vi "svx_Timebase Property Dialog.vi"(0 "Container":refnum<vi>, 1 "Data":T2, 2 "State in":T4={"X Scale"={"Name"="Time", "FString"="%#.2g", "Major Color"=16777238, "Minor Color"=16777216, "Grid Style"=1, "Maximum"=0.5, "Minimum"=0.0, "Autoscale"=TRUE, "Show Scale Label"={"Probe X"=FALSE, "Probe Y"=TRUE}, "Show Scale"={"Probe X"=TRUE, "Probe Y"=TRUE}, "Autoscale Once"=FALSE}, "Y Scale"={"Name"="Amplitude", "FString"="%#.2g", "Major Color"=16777238, "Minor Color"=16777216, "Scale Visible"=TRUE, " Label Visible"=TRUE, "Grid Style"=1, "Autoscale"=TRUE, "Maximum"={"Probe X"=1.0, "Probe Y"=1.0}, "Minimum"={"Probe X"=-1.0, "Probe Y"=-1.0}, "Autoscale Once"=FALSE}, "Plot"={"Point Style"=0, "Line Width"=0, "Line Style"=0, "Plot Color"=16860, "Point/fill"=16860}, "Tacho Point Color"=16711680, "Property Name"=[], "Container Bounds"={"Width"=640, "Height"=360}, "Background color"=16777226, "Legend Visible"=TRUE, "Scale Range Change"=refnum, "Strings[]"={"Custom pair name"=FALSE, "Row Strings []"=[], "Column Strings []"=[]}, "Cursor"={"Cursor Point Style"=13, "Cursor Style"=5, "Cursor Line Width"=1, "Cursor Line Style"=0, "Cursor Color"=16860, "Cursor Name Visible"=TRUE, "Cursor Visible"=TRUE, "Cursor Lock"=FALSE, "Cursor Index"=0}, "Index"=[], "Legend Width"=200, " Parents Tags"=[], "Children Tags"=[], "Open?"=[], "Label"="Timebase Plot", "Cursor X Pos"={"X"=0.0, "Y"=0.0}, "Cursor Y Pos"={"X"=0.0, "Y"=0.0}, "Graph Type"=enum."Probe X and Y", "Prev Graph Type"=enum."Probe X and Y", "Prev Legend Visible"=TRUE, "Cursor Release"=refnum, "Pair Strings Changed?"=FALSE, "Cursor ID"=refnum, "Legend Background"=16777226, "Legend Font"=16777222, "Probe Y Label"="Probe Y", "Probe X Label"="Probe X", "Probe X Label Visible"=TRUE, "Probe Y Label Visible"=TRUE, "Tree Item Width"=200, "# Custom RowStr"=0, "# Custom ColStr"=0, "Property Name"=refnum, "Data Related State"=refnum} caption="State", 5 "Ref Ins":T1, 7 "Facade VI":refnum<vi>, 13 "Action in":T3 caption="Action") -> (3 "State out":T4={"X Scale"={"Name"="Time", "FString"="%#.2g", "Major Color"=16777238, "Minor Color"=16777216, "Grid Style"=1, "Maximum"=0.5, "Minimum"=0.0, "Autoscale"=TRUE, "Show Scale Label"={"Probe X"=FALSE, "Probe Y"=TRUE}, "Show Scale"={"Probe X"=TRUE, "Probe Y"=TRUE}, "Autoscale Once"=FALSE}, "Y Scale"={"Name"="Amplitude", "FString"="%#.2g", "Major Color"=16777238, "Minor Color"=16777216, "Scale Visible"=TRUE, " Label Visible"=TRUE, "Grid Style"=1, "Autoscale"=TRUE, "Maximum"={"Probe X"=1.0, "Probe Y"=1.0}, "Minimum"={"Probe X"=-1.0, "Probe Y"=-1.0}, "Autoscale Once"=FALSE}, "Plot"={"Point Style"=0, "Line Width"=0, "Line Style"=0, "Plot Color"=16860, "Point/fill"=16860}, "Tacho Point Color"=16711680, "Property Name"=[], "Container Bounds"={"Width"=640, "Height"=360}, "Background color"=16777226, "Legend Visible"=TRUE, "Scale Range Change"=refnum, "Strings[]"={"Custom pair name"=FALSE, "Row Strings []"=[], "Column Strings []"=[]}, "Cursor"={"Cursor Point Style"=13, "Cursor Style"=5, "Cursor Line Width"=1, "Cursor Line Style"=0, "Cursor Color"=16860, "Cursor Name Visible"=TRUE, "Cursor Visible"=TRUE, "Cursor Lock"=FALSE, "Cursor Index"=0}, "Index"=[], "Legend Width"=200, " Parents Tags"=[], "Children Tags"=[], "Open?"=[], "Label"="Timebase Plot", "Cursor X Pos"={"X"=0.0, "Y"=0.0}, "Cursor Y Pos"={"X"=0.0, "Y"=0.0}, "Graph Type"=enum."Probe X and Y", "Prev Graph Type"=enum."Probe X and Y", "Prev Legend Visible"=TRUE, "Cursor Release"=refnum, "Pair Strings Changed?"=FALSE, "Cursor ID"=refnum, "Legend Background"=16777226, "Legend Font"=16777222, "Probe Y Label"="Probe Y", "Probe X Label"="Probe X", "Probe X Label Visible"=TRUE, "Probe Y Label Visible"=TRUE, "Tree Item Width"=200, "# Custom RowStr"=0, "# Custom ColStr"=0, "Property Name"=refnum, "Data Related State"=refnum} caption="State", 14 "Action out":T3 caption="Action")   [LabVIEW 2017, in "SVX Timebase.xctl"]
uses:
  <vilib>/addons/_XControls/Timebase Plot/SVX Timebase.xctl
  <vilib>/addons/_XControls/Timebase Plot/subVIs/svx_Timebase State.ctl
  <vilib>/addons/_XControls/Timebase Plot/subVIs/svx_Timebase Bounds.ctl
  <vilib>/addons/_XControls/Timebase Plot/subVIs/svx_Timebase Graph Types.ctl
  <vilib>/addons/_XControls/Timebase Plot/subVIs/svx_Timebase Data Related State.ctl
  <vilib>/_xctls/Action.ctl
  <vilib>/addons/_XControls/Timebase Plot/subVIs/svx_Timebase Data.ctl
  <vilib>/addons/_XControls/Timebase Plot/subVIs/svx_Timebase Core States.ctl
  <vilib>/_xctls/XControlSupport.lvlib
panel:
  in  "Help":bool
  in  "Cancel":bool
  in  "OK":bool
  in  "Main Tab":T8(tab)
  in  "Legend Font.Color":u32(colorbox)=16777222 caption="Legend font"
  in  "Legend Background.Color":u32(colorbox)=16777226 caption="Legend background"
  in  "Probe Y Label.Visible":bool=TRUE caption="Probe Y Visible"
  in  "Probe Y Label.Text":string="Probe Y"
  in  "Probe X Label.Visible":bool=TRUE caption="Probe X"
  in  "Probe X Label.Text":string="Probe X"
  in  "Background.Color":u32(colorbox)=16777226 caption="Background"
  in  "Label.Visible":bool=TRUE
  in  "Label.Text":string="Timebase Plot"
  in  "Caption.Visible":bool
  in  "Caption.Text":string="Timebase Plot"
  in  "Enable State":T9(radio)
  in  "Format Selection":u16(ring) items=["Time (X-Axis)", "Amplitude (Y-Axis)"]
  in  "Hide trailing zeros":bool=TRUE
  in  "Digits":u8=2
  in  "Precision Type":u16(ring) items=["Digits of precision", "Significant digits"]
  in  "Type":i32(listbox)=2
  in  "Point/Fill.Color":u32(colorbox) caption="Point/Fill"
  in  "Plot.Point Style":T10={"OK Button 17"=TRUE, "OK Button"=FALSE, "OK Button 2"=FALSE, "OK Button 3"=FALSE, "OK Button 4"=FALSE, "OK Button 5"=FALSE, "OK Button 6"=FALSE, "OK Button 7"=FALSE, "OK Button 8"=FALSE, "OK Button 9"=FALSE, "OK Button 10"=FALSE, "OK Button 11"=FALSE, "OK Button 12"=FALSE, "OK Button 13"=FALSE, "OK Button 14"=FALSE, "OK Button 15"=FALSE, "OK Button 16"=FALSE} caption="Point Style"
  in  "Line.Color":u32(colorbox)=9727 caption="Line"
  in  "Plot.Line Style":T11={"OK Button"=TRUE, "OK Button 2"=FALSE, "OK Button 3"=FALSE, "OK Button 4"=FALSE, "OK Button 5"=FALSE} caption="Line Style"
  in  "Plot.Line Width":T12={"OK Button 2"=TRUE, "OK Button 3"=FALSE, "OK Button 4"=FALSE, "OK Button 5"=FALSE, "OK Button 6"=FALSE, "OK Button 7"=FALSE} caption="Line Width"
  in  "Trigger Point.Color":u32(colorbox)=16711680 caption="Trigger point"
  in  "X Axis Scale":T13={"Probe Y Scale.Visible"=TRUE, "Probe Y Scale Label.Visible"=TRUE, "Probe X Scale.Visible"=TRUE, "Probe X Scale Label.Visible"=TRUE}
  in  "X Axis Range":cluster{"Minimum X":dbl, "Maximum X":dbl}={"Minimum X"=0.0, "Maximum X"=0.5} {"Maximum X" format="%#.6g"; "Minimum X" format="%#.6g"}
  in  "Y Axis Scale":T14={"Scale Visible"=TRUE, "Scale Label Visible"=TRUE}
  in  "Y Axis Range":T15={"Minimum Y [Probe X]"=0.0, "Maximum Y [Probe X]"=10.0, "Minimum Y [Probe Y]"=0.0, "Maximum Y [Probe Y]"=10.0} {"Maximum Y [Probe Y]" format="%#.6g"; "Minimum Y [Probe Y]" format="%#.6g"; "Maximum Y [Probe X]" format="%#.6g"; "Minimum Y [Probe X]" format="%#.6g"}
  in  "YGrid Style":u16(ring) caption="Grid Style and Colors"
  in  "XGrid Style":u16(ring)=1 caption="Grid Style and Colors"
  in  "Minor Grid.Color":u32(colorbox)=16777216 caption="Minor grid"
  in  "Major Grid.Color":u32(colorbox)=16777238 caption="Major grid"
  in  "Scale Fit":bool=TRUE caption="Autoscale"
  in  "Scale Name":string="Time" caption="Name"
  in  "Scale Selection":u16(ring) items=["Time (X-Axis)", "Amplitude (Y-Axis)"]
  in  "Cursor Info Position.Lock":bool
  in  "Cursor.Line Width":T12={"OK Button 2"=FALSE, "OK Button 3"=TRUE, "OK Button 4"=FALSE, "OK Button 5"=FALSE, "OK Button 6"=FALSE, "OK Button 7"=FALSE} caption="Cursor Line Width"
  in  "Cursor.Point Style":T10={"OK Button 17"=FALSE, "OK Button"=FALSE, "OK Button 2"=FALSE, "OK Button 3"=FALSE, "OK Button 4"=FALSE, "OK Button 5"=FALSE, "OK Button 6"=FALSE, "OK Button 7"=FALSE, "OK Button 8"=FALSE, "OK Button 9"=FALSE, "OK Button 10"=FALSE, "OK Button 11"=FALSE, "OK Button 12"=FALSE, "OK Button 13"=TRUE, "OK Button 14"=FALSE, "OK Button 15"=FALSE, "OK Button 16"=FALSE} caption="Cursor Point Style"
  in  "Cursor.Line Style":T11={"OK Button"=TRUE, "OK Button 2"=FALSE, "OK Button 3"=FALSE, "OK Button 4"=FALSE, "OK Button 5"=FALSE} caption="Cursor Line Style"
  in  "Cursor Info.Visible":bool=TRUE caption="Show name"
  in  "Cursor.Style":T16={"OK Button 17"=FALSE, "OK Button"=FALSE, "OK Button 2"=FALSE, "OK Button 5"=FALSE, "OK Button 13"=FALSE, "OK Button 10"=TRUE, "OK Button 6"=FALSE, "OK Button 9"=FALSE, "OK Button 14"=FALSE} caption="Cursor Style"
  in  "Cursor.Color":u32(colorbox)=9727 caption="Cursor color"
  in  "Cursor.Visible":bool=TRUE
  in  "Tip strip":string
  in  "Description":string
  # "Label"
  # "Caption"
  # "Probe X Label"
  # "Probe Y Label"
  # "Color Scheme"
  # "Enabled State"
  # "Timebase Plot"
  # "Colors"
  # "Cursor"
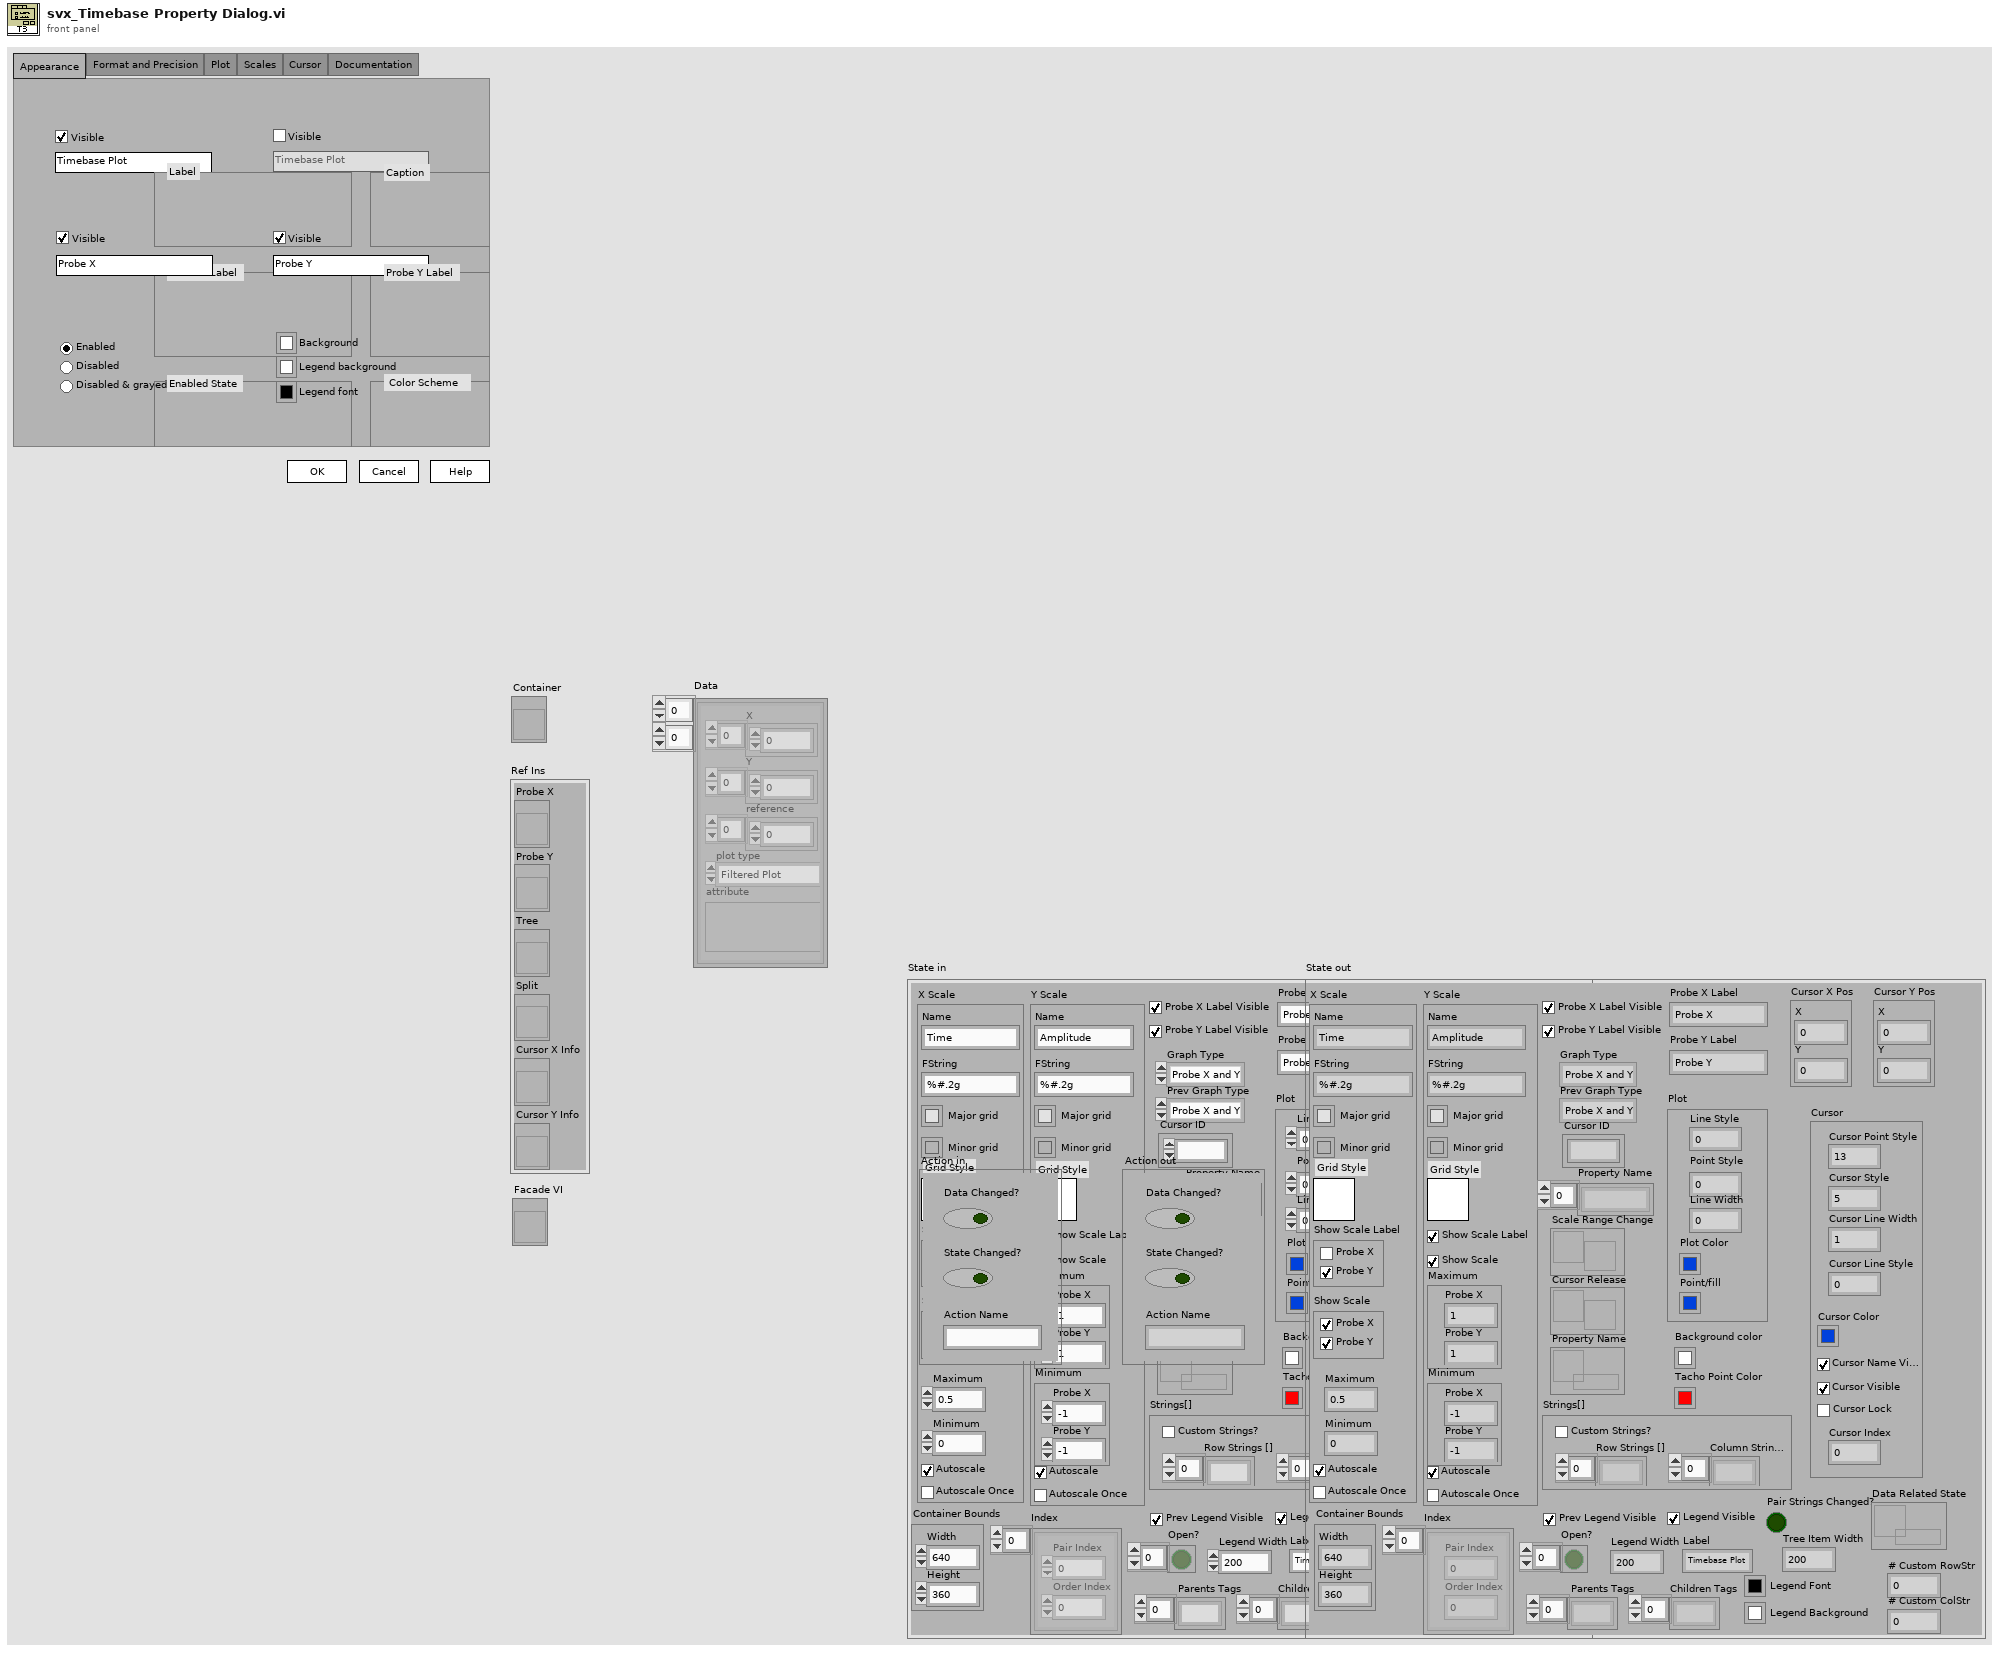
[diagram p1: front panel]
types:
  T1 = cluster{"Probe X":refnum<vi>, "Probe Y":refnum<vi>, "Tree":refnum<vi>, "Split":refnum<vi>, "Cursor X Info":refnum<vi>, "Cursor Y Info":refnum<vi>}
  T2 = typedef "SVX Timebase.xctl/svx_Timebase Data.ctl" = cluster{"X":dbl[], "Y":dbl[], "reference":dbl[], "plot type":enum16{"Filtered Plot", "Unfiltered Plot"}, "attribute":variant}[][]
  T3 = typedef "XControlSupport.lvlib/Action.ctl" = cluster{"Data Changed?":bool, "State Changed?":bool, "Action Name":string}
  T4 = typedef "SVX Timebase.xctl/svx_Timebase State.ctl" = cluster{"X Scale":cluster{"Name":string, "FString":string, "Major Color":u32, "Minor Color":u32, "Grid Style":u16, "Maximum":dbl, "Minimum":dbl, "Autoscale":bool, "Show Scale Label":cluster{"Probe X":bool, "Probe Y":bool}, "Show Scale":cluster{"Probe X":bool, "Probe Y":bool}, "Autoscale Once":bool}, "Y Scale":cluster{"Name":string, "FString":string, "Major Color":u32, "Minor Color":u32, "Scale Visible":bool, " Label Visible":bool, "Grid Style":u16, "Autoscale":bool, "Maximum":cluster{"Probe X":dbl, "Probe Y":dbl}, "Minimum":cluster{"Probe X":dbl, "Probe Y":dbl}, "Autoscale Once":bool}, "Plot":cluster{"Point Style":u8, "Line Width":u8, "Line Style":u8, "Plot Color":u32, "Point/fill":u32}, "Tacho Point Color":u32, "Property Name":string[], "Container Bounds":T5, "Background color":u32, "Legend Visible":bool, "Scale Range Change":refnum<user-event>, "Strings[]":cluster{"Custom pair name":bool, "Row Strings []":string[], "Column Strings []":string[]}, "Cursor":cluster{"Cursor Point Style":u8, "Cursor Style":u8, "Cursor Line Width":u8, "Cursor Line Style":u8, "Cursor Color":u32, "Cursor Name Visible":bool, "Cursor Visible":bool, "Cursor Lock":bool, "Cursor Index":i32}, "Index":cluster{"Pair Index":u32, "Order Index":u32}[], "Legend Width":u32, " Parents Tags":string[], "Children Tags":string[], "Open?":bool[], "Label":string, "Cursor X Pos":cluster{"X":dbl, "Y":dbl}, "Cursor Y Pos":cluster{"X":dbl, "Y":dbl}, "Graph Type":T6, "Prev Graph Type":T6, "Prev Legend Visible":bool, "Cursor Release":refnum<user-event>, "Pair Strings Changed?":bool, "Cursor ID":refnum<k1>, "Legend Background":u32, "Legend Font":u32, "Probe Y Label":string, "Probe X Label":string, "Probe X Label Visible":bool, "Probe Y Label Visible":bool, "Tree Item Width":u32, "# Custom RowStr":u32, "# Custom ColStr":u32, "Property Name":refnum<queue>, "Data Related State":T7}
  T5 = typedef "SVX Timebase.xctl/svx_Timebase Bounds.ctl" = cluster{"Width":u32, "Height":u32}
  T6 = typedef "SVX Timebase.xctl/svx_Timebase Graph Types.ctl" = enum16{"Probe X", "Probe Y", "Probe X and Y"}
  T7 = typedef "SVX Timebase.xctl/svx_Timebase Data Related State.ctl" = refnum<queue>
  T8 = enum32{"Appearance", "Format and Precision", "Plot", "Scales", "Cursor", "Documentation"}
  T9 = enum32{"Enabled", "Disabled", "Disabled & grayed"}
  T10 = cluster{"OK Button 17":bool, "OK Button":bool, "OK Button 2":bool, "OK Button 3":bool, "OK Button 4":bool, "OK Button 5":bool, "OK Button 6":bool, "OK Button 7":bool, "OK Button 8":bool, "OK Button 9":bool, "OK Button 10":bool, "OK Button 11":bool, "OK Button 12":bool, "OK Button 13":bool, "OK Button 14":bool, "OK Button 15":bool, "OK Button 16":bool}
  T11 = cluster{"OK Button":bool, "OK Button 2":bool, "OK Button 3":bool, "OK Button 4":bool, "OK Button 5":bool}
  T12 = cluster{"OK Button 2":bool, "OK Button 3":bool, "OK Button 4":bool, "OK Button 5":bool, "OK Button 6":bool, "OK Button 7":bool}
  T13 = cluster{"Probe Y Scale.Visible":bool, "Probe Y Scale Label.Visible":bool, "Probe X Scale.Visible":bool, "Probe X Scale Label.Visible":bool}
  T14 = cluster{"Scale Visible":bool, "Scale Label Visible":bool}
  T15 = cluster{"Minimum Y [Probe X]":dbl, "Maximum Y [Probe X]":dbl, "Minimum Y [Probe Y]":dbl, "Maximum Y [Probe Y]":dbl}
  T16 = cluster{"OK Button 17":bool, "OK Button":bool, "OK Button 2":bool, "OK Button 5":bool, "OK Button 13":bool, "OK Button 10":bool, "OK Button 6":bool, "OK Button 9":bool, "OK Button 14":bool}
  T17 = cluster{"Desc":string, "TipStrip":string, "Label.Text":string, "Label.Visible":bool, "Caption.Text":string, "Caption.Visible":bool, "Disabled":u8}
  T18 = cluster{"X":dbl[], "Y":dbl[], "reference":dbl[], "plot type":enum16{"Filtered Plot", "Unfiltered Plot"}, "attribute":variant}
  T19 = typedef "SVX Timebase.xctl/svx_Timebase Core States.ctl" = enum16{"None", "[Axis] Range X Scale", "[Axis] Range Y Scale", "[Layout] Graph Type Change", "[Plot] Tacho Point", "[Plot] Grid and BG", "[Cursor] Cursor Info", "[Legend] Pair Strings", "[Data] Plot Data", "[Legend] Checkbox", "[Layout] Update", "[Legend] Tree Open", "[Layout] Legend Visible Change", "[Plot] Data Point", "[Cursor] Appearance", "[Cursor] Index", "[Legend] Color", "[Axis] Axis and Label", "[Axis] Format String", "[Layout] Min Pane Size", "[Data] Index", "[Plot] Caption", "[Data] Legend Strings"}
  T20 = cluster{"Probe X":dbl, "Probe X":dbl, "Probe Y":dbl, "Probe Y":dbl}
  T21 = cluster{"Scale Visible":bool, " Label Visible":bool}
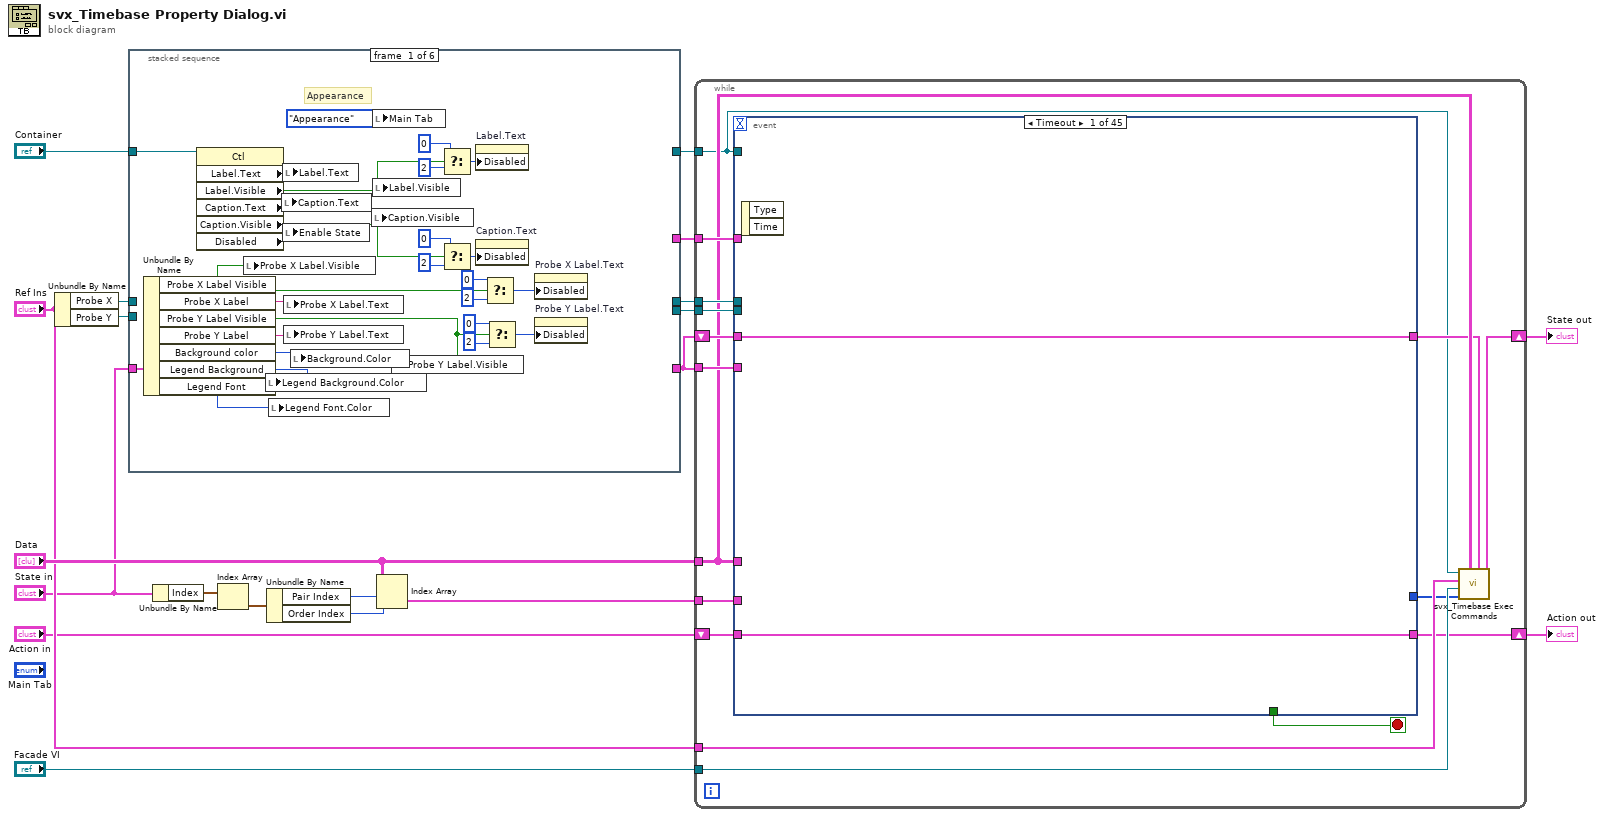
[diagram p0: block diagram]
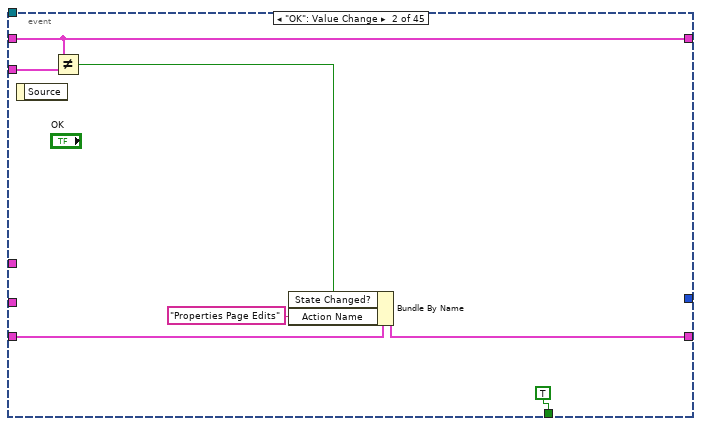
[diagram p2: hidden frame]
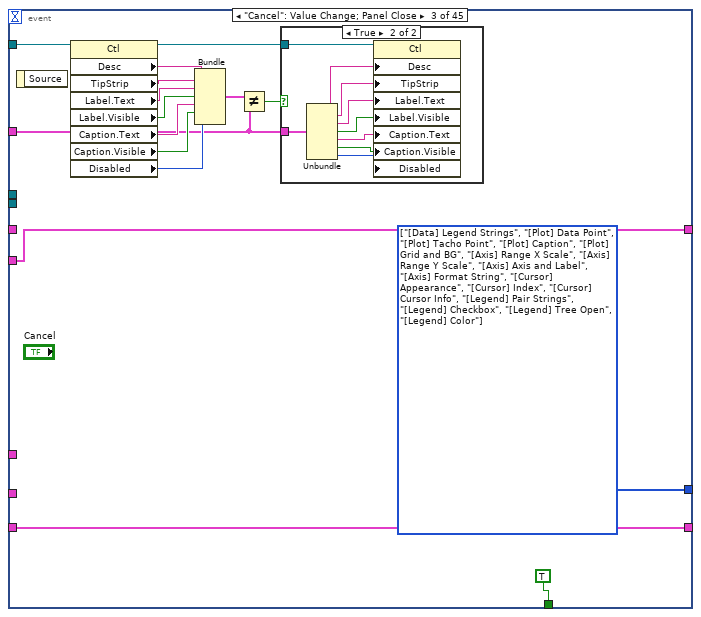
[diagram p3: hidden frame]
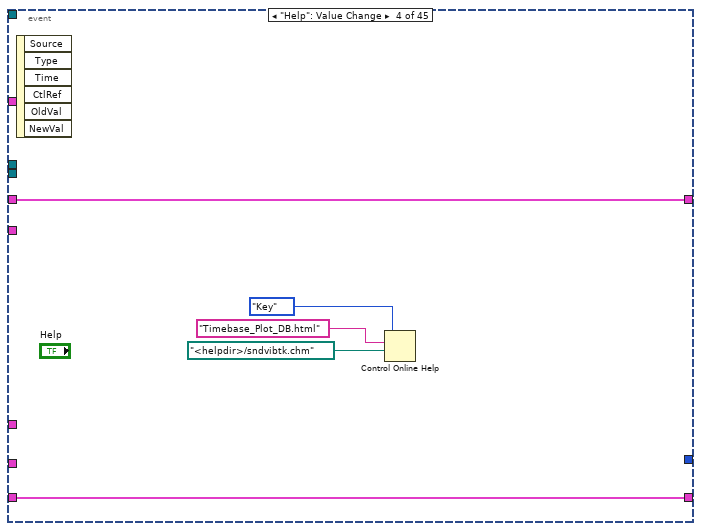
[diagram p5: hidden frame]
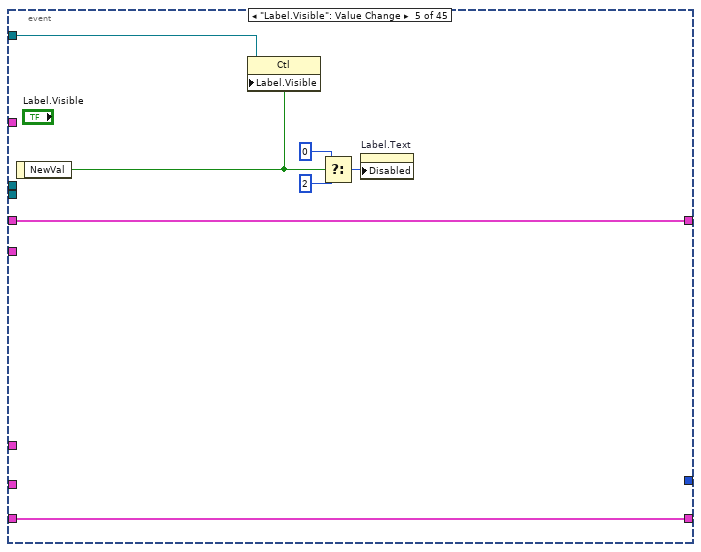
[diagram p6: hidden frame]
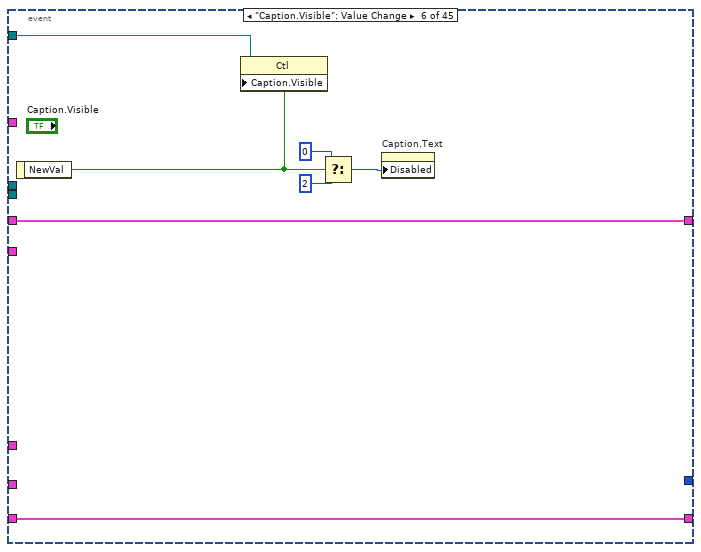
[diagram p7: hidden frame]
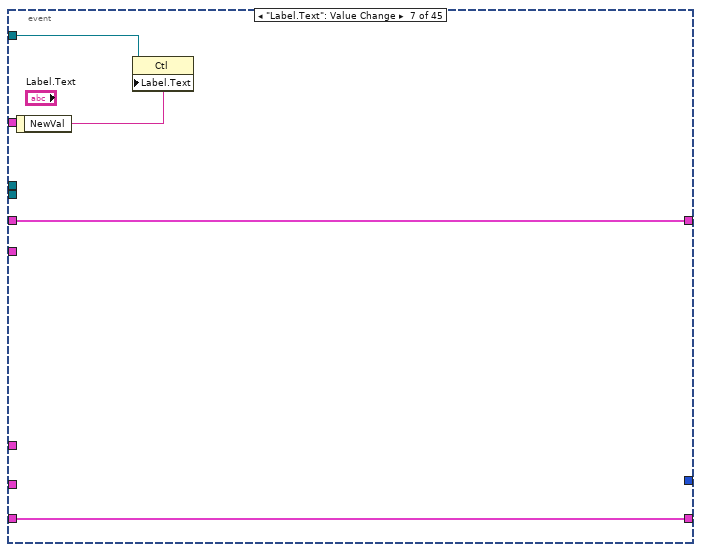
[diagram p8: hidden frame]
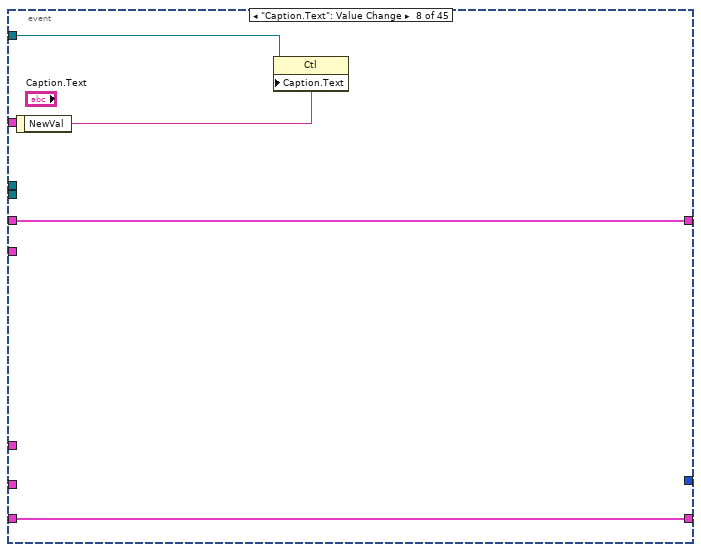
[diagram p9: hidden frame]
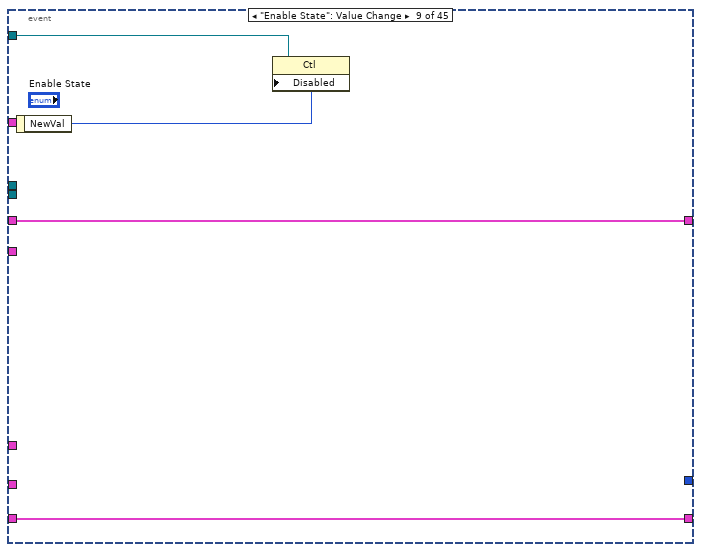
[diagram p10: hidden frame]
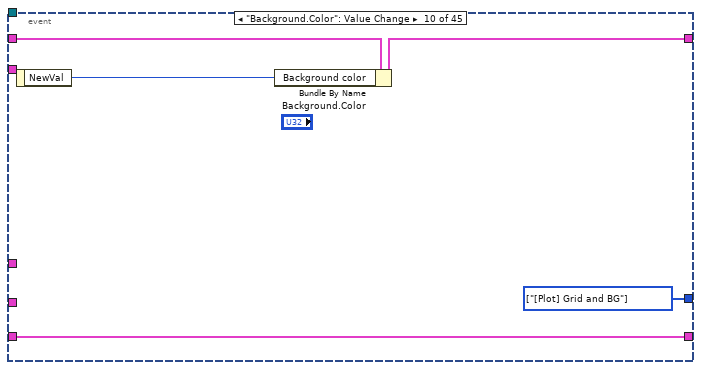
[diagram p11: hidden frame]
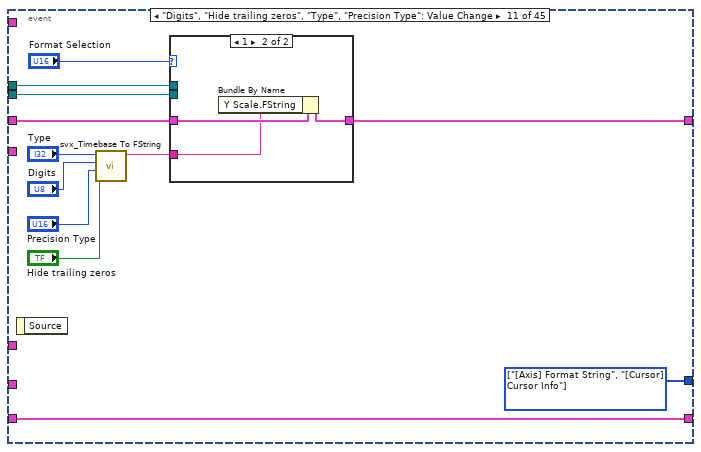
[diagram p12: hidden frame]
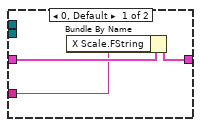
[diagram p13: hidden frame]
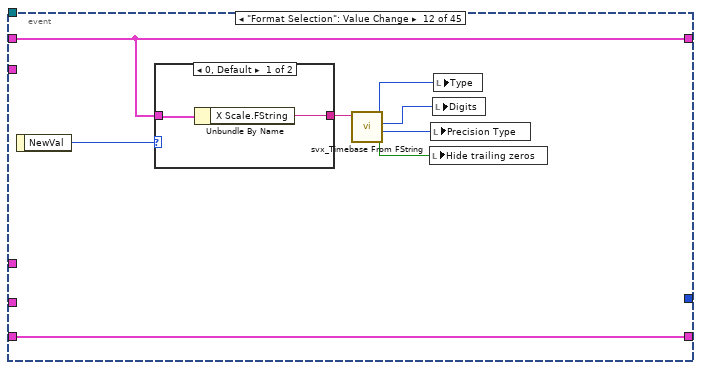
[diagram p14: hidden frame]
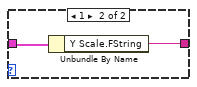
[diagram p15: hidden frame]
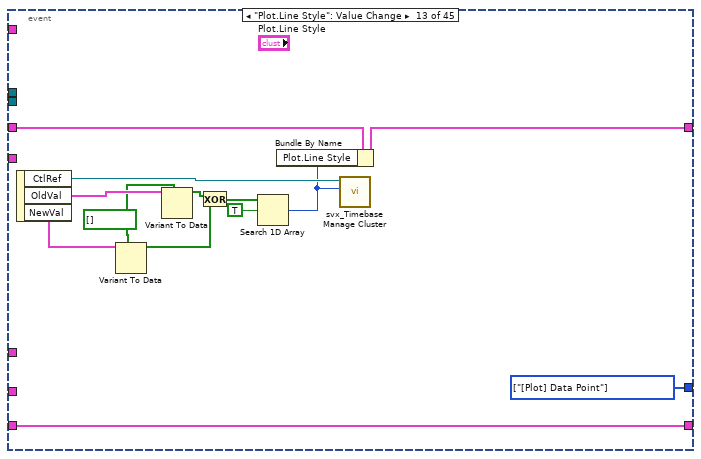
[diagram p16: hidden frame]
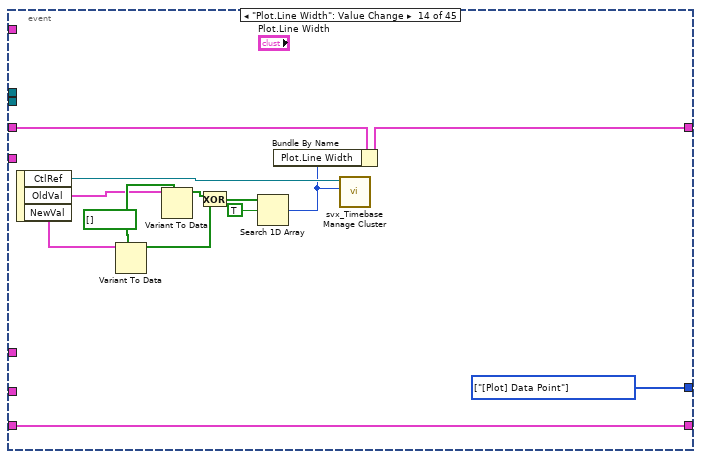
[diagram p17: hidden frame]
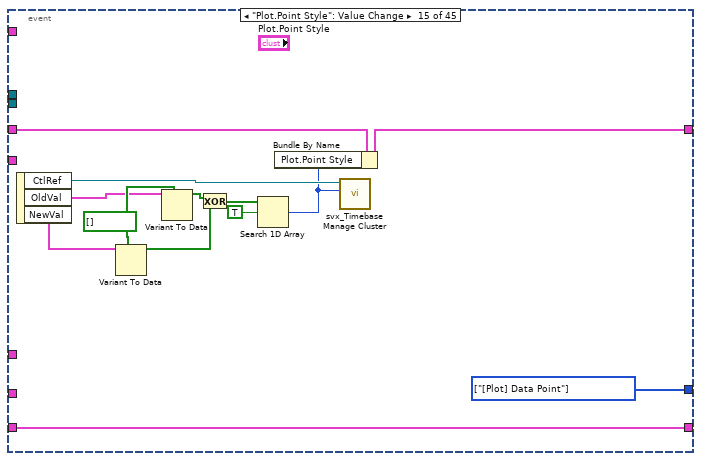
[diagram p18: hidden frame]
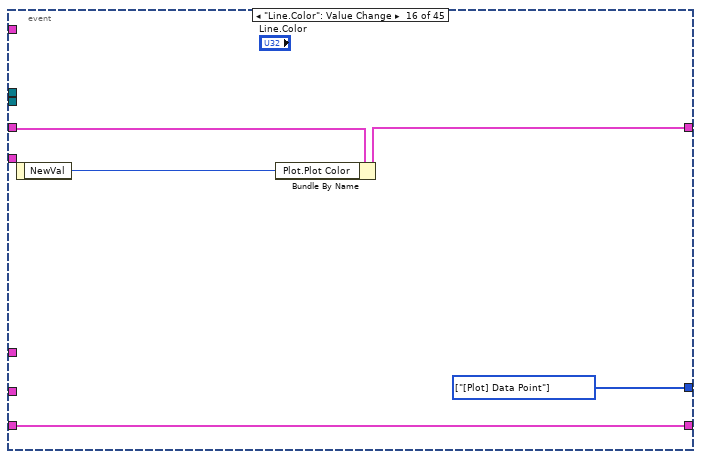
[diagram p19: hidden frame]
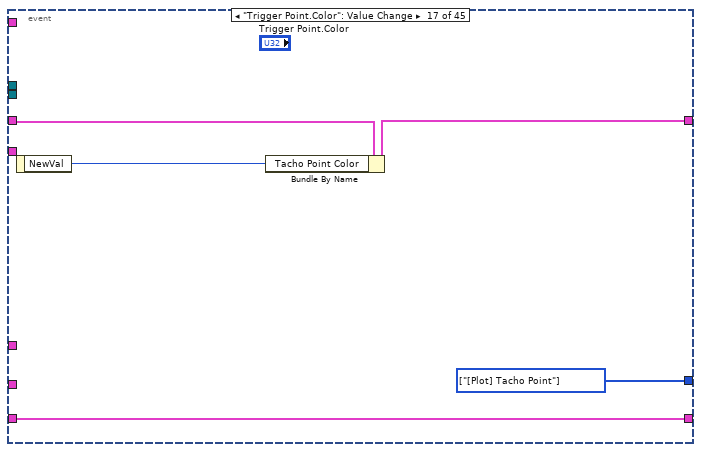
[diagram p20: hidden frame]
diagram:
  n1 = Unbundle By Name("Ref Ins") -> ("Probe X"=w6:refnum<vi>, "Probe Y"=w5:refnum<vi>)
  n2 = stacked-sequence {
    tunnel: "Container" -> [w47 _ _ _ _ w145]
    tunnel: "State in" -> [w45 w60 w74 w101 w132 w135]
    tunnel: [_ _ _ _ _ w144] -> w19
    tunnel: [_ _ _ _ _ w135] -> w18
    tunnel: [_ _ _ _ _ w134] -> w16
    tunnel: w6 -> [_ _ _ _ _ w134]
    tunnel: [_ _ _ _ _ w136] -> w15
    tunnel: w5 -> [_ _ _ _ _ w133]
    tunnel: [_ _ _ _ _ w133] -> w7
    frame #0 {
      # "Appearance"
      n3 = Unbundle By Name(w45) -> ("Probe X Label Visible"=w28:bool, "Probe X Label"=w32:string, "Probe Y Label Visible"=w24:bool, "Probe Y Label"=w31:string, "Background color"=w46:u32, "Legend Background"=w22:u32, "Legend Font"=w21:u32)
      n4 = property class="Ctl"(reference=w47) -> ("Label.Text"=w39:string, "Label.Visible"=w38:bool, "Caption.Text"=w37:string, "Caption.Visible"=w35:bool, "Disabled"=w36:u8)  [unwired: 1 in, 2 out]
      n5 = local write "Probe X Label.Visible"(w28) -> ()
      n6 = local write "Legend Background.Color"(w22) -> ()
      n7 = local write "Legend Font.Color"(w21) -> ()
      n8 = local write "Caption.Text"(w37) -> ()
      n9 = local write "Label.Text"(w39) -> ()
      n10 = local write "Enable State"(w36) -> ()
      n11 = local write "Probe X Label.Text"(w32) -> ()
      n12 = local write "Probe Y Label.Text"(w31) -> ()
      n13 = local write "Background.Color"(w46) -> ()
      n14 = local write "Caption.Visible"(w35) -> ()
      n15 = local write "Main Tab"(T8."Appearance" ("Main Tab")) -> ()
      n16 = local write "Label.Visible"(w38) -> ()
      n17 = local write "Probe Y Label.Visible"(w24) -> ()
      n18 = Select(t=u8 0 ("Disabled"), s=w38, f=u8 2) -> (s? t:f=w43:u8)
      n19 = Select(t=u8 0 ("Disabled"), s=w35, f=u8 2) -> (s? t:f=w40:u8)
      n20 = property on="Label.Text" class="Str"("Disabled"=w43) -> ()  [unwired: 2 in, 2 out]
      n21 = property on="Caption.Text" class="Str"("Disabled"=w40) -> ()  [unwired: 2 in, 2 out]
      n22 = Select(t=u8 0 ("Disabled"), s=w28, f=u8 2) -> (s? t:f=w27:u8)
      n23 = Select(t=u8 0 ("Disabled"), s=w24, f=u8 2) -> (s? t:f=w23:u8)
      n24 = property on="Probe X Label.Text" class="Str"("Disabled"=w27) -> ()  [unwired: 2 in, 2 out]
      n25 = property on="Probe Y Label.Text" class="Str"("Disabled"=w23) -> ()  [unwired: 2 in, 2 out]
    }
    frame #1 {
      w61 = u16 0 items=["X-Axis", "Y-Axis"] ("Format selection")
      # "On Tab 3"
      # "Format and Precision"
      n26 = Unbundle By Name(w60) -> ("X Scale.Name"=w54:string, "Y Scale.Name"=w51:string, "X Scale.FString"=w59:string)
      n27 = call <vilib>:"svx_Timebase From FString.vi"("Format string"=w59) -> ("trailing zeros"=w55:bool, "Precision Type"=w56:u16, "Digits"=w57:u8, "Type"=w58:i32)  [unwired: 7 in]
      n28 = local write "Format Selection"(w61) -> ()
      n29 = Concatenate Strings(w54, " (X-Axis)" ("string")) -> (w50:string)
      n30 = Concatenate Strings(w51, " (Y-Axis)" ("string")) -> (w49:string)
      n31 = local write "Hide trailing zeros"(w55) -> ()
      n32 = local write "Precision Type"(w56) -> ()
      n33 = local write "Digits"(w57) -> ()
      n34 = local write "Type"(w58) -> ()
      n35 = Build Array(w50, w49) -> (w48:string[])
      n36 = property on="Format Selection" class="Ring (strict)"("Strings []"=w48) -> ()  [unwired: 2 in, 2 out]
      n37 = property on="Scale Selection" class="Ring (strict)"("Strings []"=w48) -> ()  [unwired: 2 in, 2 out]
    }
    frame #2 {
      # "Plot"
      n38 = Unbundle By Name(w74) -> ("Plot.Plot Color"=w67:u32, "Tacho Point Color"=w66:u32, "Plot.Point/fill"=w65:u32, "Plot.Line Width"=w73:u8, "Plot.Line Style"=w71:u8, "Plot.Point Style"=w70:u8)
      n39 = control-ref of="Plot.Line Width"() -> (w72:refnum<vi>)
      n40 = control-ref of="Plot.Line Style"() -> (w68:refnum<vi>)
      n41 = control-ref of="Plot.Point Style"() -> (w69:refnum<vi>)
      n42 = To Long Integer(number=w73) -> (32bit integer=w64:i32)
      n43 = To Long Integer(number=w71) -> (32bit integer=w63:i32)
      n44 = To Long Integer(number=w70) -> (32bit integer=w62:i32)
      n45 = local write "Point/Fill.Color"(w65) -> ()
      n46 = local write "Trigger Point.Color"(w66) -> ()
      n47 = local write "Line.Color"(w67) -> ()
      n48 = call <vilib>:"svx_Timebase Manage Cluster.vi"("index"=w64, "Cursor Refnum"=w72) -> ()  [unwired: 10 in]
      n49 = call <vilib>:"svx_Timebase Manage Cluster.vi"("index"=w63, "Cursor Refnum"=w68) -> ()  [unwired: 10 in]
      n50 = call <vilib>:"svx_Timebase Manage Cluster.vi"("index"=w62, "Cursor Refnum"=w69) -> ()  [unwired: 10 in]
    }
    frame #3 {
      w102 = u16 0 items=["X-Axis", "Y-Axis"] ("Scale selection")
      # "Scales"
      n51 = Unbundle By Name(w101) -> ("X Scale.Name"=w100:string, "X Scale.Show Scale.Probe X"=w78:bool, "X Scale.Show Scale Label.Probe X"=w77:bool, "X Scale.Show Scale.Probe Y"=w76:bool, "X Scale.Show Scale Label.Probe Y"=w75:bool, "X Scale.Grid Style"=w91:u16, "X Scale.Major Color"=w99:u32, "X Scale.Minor Color"=w98:u32, "X Scale.Autoscale"=w95:bool, "X Scale.Minimum"=w87:dbl, "X Scale.Maximum"=w86:dbl)
      n52 = property on="YGrid Style" class="Ring (strict)"("Visible"=FALSE) -> ()  [unwired: 2 in, 2 out]
      n53 = property on="XGrid Style" class="Ring (strict)"("Visible"=TRUE) -> ()  [unwired: 2 in, 2 out]
      n54 = Bundle("Minimum"=w87, "Maximum"=w86) -> (w85:cluster{"Minimum":dbl, "Maximum":dbl})  [unwired: 1 in]
      n55 = local write "X Axis Range"(w85) -> ()
      n56 = local write "Scale Selection"(w102) -> ()
      n57 = local write "Minor Grid.Color"(w98) -> ()
      n58 = local write "XGrid Style"(w91) -> ()
      n59 = case shown="0, Default" w91 {
        tunnel: [w105 u8 0 ("Disabled") w108] -> w93
        tunnel: [w105 u8 2 ("Disabled") w108] -> w92
        frame 0, Default {
          w105 = u8 2 ("Disabled")
        }
        frame 1 {
        }
        frame 2 {
          w108 = u8 0 ("Disabled")
        }
      }
      n60 = local write "Scale Name"(w100) -> ()
      n61 = Select(t=u8 2 ("Disabled"), s=w95, f=u8 0) -> (s? t:f=w83:u8)
      n62 = property on="X Axis Range" class="Clust (strict)"("Disabled"=w83, "Visible"=TRUE) -> ("Controls[]"=w84:refnum<vi>[])  [unwired: 2 in, 2 out]
      n63 = Bundle By Name(cluster=T13 {"Probe Y Scale.Visible"=TRUE, "Probe Y Scale Label.Visible"=TRUE, "Probe X Scale.Visible"=TRUE, "Probe X Scale Label.Visible"=TRUE} ("X Axis Scale"), "Probe X Scale.Visible"=w78, "Probe X Scale Label.Visible"=w77, "Probe Y Scale.Visible"=w76, "Probe Y Scale Label.Visible"=w75) -> (w79:T13)
      n64 = local write "Major Grid.Color"(w99) -> ()
      n65 = local write "Scale Fit"(w95) -> ()
      n66 = property on="Major Grid.Color" class="ColBox"("Disabled"=w93) -> ()  [unwired: 2 in, 2 out]
      n67 = property on="Minor Grid.Color" class="ColBox"("Disabled"=w92) -> ()  [unwired: 2 in, 2 out]
      n68 = for {
        tunnel: w84 -> [w104] mode=indexing
        tunnel: w83 -> [w103]
        n69 = property class="Ctl"(reference=w104, "Disabled"=w103) -> ()  [unwired: 1 in, 2 out]
      }
      n70 = property on="Y Axis Range" class="Clust (strict)"("Visible"=FALSE) -> ()  [unwired: 2 in, 2 out]
      n71 = property on="X Axis Scale" class="Clust (strict)"("Visible"=TRUE) -> ()  [unwired: 2 in, 2 out]
      n72 = property on="Y Axis Scale" class="Clust (strict)"("Visible"=FALSE) -> ()  [unwired: 2 in, 2 out]
      n73 = local write "X Axis Scale"(w79) -> ()
    }
    frame #4 {
      # "Cursor"
      n74 = Unbundle By Name(w132) -> ("Cursor.Cursor Point Style"=w131:u8, "Cursor.Cursor Style"=w129:u8, "Cursor.Cursor Line Width"=w127:u8, "Cursor.Cursor Line Style"=w125:u8, "Cursor.Cursor Color"=w123:u32, "Cursor.Cursor Lock"=w122:bool, "Cursor.Cursor Name Visible"=w115:bool, "Cursor.Cursor Visible"=w114:bool)
      n75 = control-ref of="Cursor.Point Style"() -> (w130:refnum<vi>)
      n76 = local write "Cursor.Visible"(w114) -> ()
      n77 = To Long Integer(number=w131) -> (32bit integer=w109:i32)
      n78 = local write "Cursor Info.Visible"(w115) -> ()
      n79 = local write "Cursor Info Position.Lock"(w122) -> ()
      n80 = call <vilib>:"svx_Timebase Manage Cluster.vi"("index"=w109, "Cursor Refnum"=w130) -> ()  [unwired: 10 in]
      n81 = And(x=w115, y=w114) -> (x .and. y?=w113:bool)
      n82 = To Long Integer(number=w129) -> (32bit integer=w112:i32)
      n83 = To Long Integer(number=w125) -> (32bit integer=w110:i32)
      n84 = control-ref of="Cursor.Style"() -> (w128:refnum<vi>)
      n85 = control-ref of="Cursor.Line Style"() -> (w124:refnum<vi>)
      n86 = local write "Cursor.Color"(w123) -> ()
      n87 = To Long Integer(number=w127) -> (32bit integer=w111:i32)
      n88 = call <vilib>:"svx_Timebase Manage Cluster.vi"("index"=w112, "Cursor Refnum"=w128) -> ()  [unwired: 10 in]
      n89 = call <vilib>:"svx_Timebase Manage Cluster.vi"("index"=w110, "Cursor Refnum"=w124) -> ()  [unwired: 10 in]
      n90 = Select(t=u8 0, s=w113, f=u8 2) -> (s? t:f=w116:u8)
      n91 = Select(t=u8 0, s=w114, f=u8 2) -> (s? t:f=w121:u8)
      n92 = control-ref of="Cursor.Line Width"() -> (w126:refnum<vi>)
      n93 = property on="Cursor Info Position.Lock" class="Bool (strict)"("Disabled"=w116) -> ()  [unwired: 2 in, 2 out]
      n94 = property on="Cursor Info.Visible" class="Bool (strict)"("Disabled"=w121) -> ()  [unwired: 2 in, 2 out]
      n95 = call <vilib>:"svx_Timebase Manage Cluster.vi"("index"=w111, "Cursor Refnum"=w126) -> ()  [unwired: 10 in]
    }
    frame #5 {
      n96 = property class="Ctl"(reference=w145) -> (reference out=w144:refnum<vi>, "Desc"=w137:string, "TipStrip"=w138:string, "Label.Text"=w143:string, "Label.Visible"=w142:bool, "Caption.Text"=w141:string, "Caption.Visible"=w140:bool, "Disabled"=w139:u8)  [unwired: 1 in, 1 out]
      n97 = local write "Description"(w137) -> ()
      n98 = local write "Tip strip"(w138) -> ()
      n99 = Bundle("Desc"=w137, "TipStrip"=w138, "Label.Text"=w143, "Label.Visible"=w142, "Caption.Text"=w141, "Caption.Visible"=w140, "Disabled"=w139) -> (w136:T17)  [unwired: 1 in]
    }
  }
  n100 = Unbundle By Name("State in") -> ("Index"=w11:cluster{"Pair Index":u32, "Order Index":u32}[])
  n101 = Index Array(array=w11) -> (element=w10:cluster{"Pair Index":u32, "Order Index":u32})  [unwired: 1 in]
  n102 = Unbundle By Name(w10) -> ("Pair Index"=w9:u32, "Order Index"=w8:u32)
  n103 = Index Array(array="Data", index (row)=w9, index (col)=w8) -> (element=w12:T18)
  n104 = while {
    tunnel: w19 -> [w149]
    shift-right: [w152] -> w14
    shift-left: w18 -> [w160]
    tunnel: w18 -> [w157]
    tunnel: w16 -> [w159]
    tunnel: w15 -> [w158]
    tunnel: "Data" -> [w154]
    tunnel: w12 -> [w156]
    tunnel: w7 -> [w155]
    tunnel: "Ref Ins" -> [w151]
    tunnel: "Facade VI" -> [w150]
    shift-right: [w146] -> w17
    shift-left: "Action in" -> [w148]
    stop <- w161 stop-if-true
    n105 = event shown="[0] Timeout" {
      selector: _ -> [_ _ _ _ _ _ _ _ _ _ _ _ _ _ _ _ _ _ _ _ _ _ _ _ _ _ _ _ _ _ _ _ _ _ _ _ _ _ _ _ _ _ _ _ _]
      dyn-events: _ -> [_ _ _ _ _ _ _ _ _ _ _ _ _ _ _ _ _ _ _ _ _ _ _ _ _ _ _ _ _ _ _ _ _ _ _ _ _ _ _ _ _ _ _ _ _]
      timeout: _ -> [_ _ _ _ _ _ _ _ _ _ _ _ _ _ _ _ _ _ _ _ _ _ _ _ _ _ _ _ _ _ _ _ _ _ _ _ _ _ _ _ _ _ _ _ _]
      tunnel: [_ TRUE TRUE _ _ _ _ _ _ _ _ _ _ _ _ _ _ _ _ _ _ _ _ _ _ _ _ _ _ _ _ _ _ _ _ _ _ _ _ _ _ _ _ _ _] -> w161
      tunnel: w160 -> [w163 w165 _ w200 w202 w209 w215 w220 w224 w231 w237 w256 w266 w282 w295 w305 w310 w319 w325 w329 w336 w359 w368 w411 w417 w428 w439 w451 w465 w522 w535 w548 w561 w574 w579 w584 w589 w602 w610 w618 w626 w631 w636 w641 w645]
      tunnel: w157 -> [_ w164 w184 _ _ _ _ _ _ _ _ _ _ _ _ _ _ _ _ _ _ _ _ _ _ _ _ _ _ _ _ _ _ _ _ _ _ _ _ _ _ _ _ _ _]
      tunnel: w148 -> [w162 w169 w186 w199 w201 w208 w216 w219 w223 w227 w232 w250 w262 w275 w288 w301 w306 w311 w324 w328 w332 w354 w360 w403 w412 w423 w434 w446 w458 w515 w528 w541 w554 w567 w575 w580 w585 w590 w603 w611 w619 w627 w632 w637 w642]
      tunnel: [w162 w168 w186 w199 w201 w208 w216 w219 w223 w227 w232 w250 w262 w275 w288 w301 w306 w311 w324 w328 w332 w354 w360 w403 w412 w423 w434 w446 w458 w515 w528 w541 w554 w567 w575 w580 w585 w590 w603 w611 w619 w627 w632 w637 w642] -> w146
      tunnel: [_ _ w183 _ _ _ _ _ _ w228 w233 _ w263 w276 w289 w302 w307 w312 _ _ w333 w355 _ w404 w416 w427 w435 w447 _ w516 w529 w542 w555 w568 w576 w581 w586 w591 w604 w612 w620 w628 w633 w638 w643] -> w147
      tunnel: w159 -> [_ _ _ _ _ _ _ _ _ _ w235 _ _ _ _ _ _ _ _ _ _ _ w369 _ _ _ _ _ _ _ _ _ _ _ _ _ _ _ _ _ _ _ _ _ _]
      tunnel: w149 -> [_ _ w182 _ w207 w214 w218 w222 w226 _ _ _ _ _ _ _ _ _ w327 w331 _ _ _ _ _ _ _ _ _ _ _ _ _ _ _ _ _ _ _ _ _ _ _ _ _]
      tunnel: w158 -> [_ _ w172 _ _ _ _ _ _ _ _ _ _ _ _ _ _ _ _ _ _ _ _ _ _ _ _ _ _ _ _ _ _ _ _ _ _ _ _ _ _ _ _ _ _]
      tunnel: [w163 w165 w184 w200 w202 w209 w215 w220 w224 w230 w236 w256 w265 w281 w294 w304 w308 w323 w325 w329 w335 w358 w365 w410 w418 w429 w438 w450 w465 w521 w534 w547 w560 w573 w577 w582 w588 w601 w609 w617 w625 w630 w635 w640 w644] -> w153
      tunnel: w154 -> [_ _ _ _ _ _ _ _ _ _ _ _ _ _ _ _ _ _ _ _ _ _ _ _ _ _ _ _ _ _ _ _ _ _ _ _ _ _ _ _ _ _ _ _ _]
      tunnel: w156 -> [_ _ _ _ _ _ _ _ _ _ _ _ _ _ _ _ _ _ _ _ _ _ w364 _ _ _ _ _ _ _ _ _ _ _ _ _ _ _ _ _ _ _ _ _ _]
      tunnel: w155 -> [_ _ _ _ _ _ _ _ _ _ w234 _ _ _ _ _ _ _ _ _ _ _ w362 _ _ _ _ _ _ _ _ _ _ _ _ _ _ _ _ _ _ _ _ _ _]
      event Timeout {
        n106 = event-data() -> ()  [unwired: 1 in, 2 out]
      }
      event "OK": Value Change {
        n107 = event-data() -> ()  [unwired: 1 in, 1 out]
        n108 = Not Equal?(x=w165, y=w164) -> (x != y?=w167:bool)
        n109 = Bundle By Name(cluster=w169, "State Changed?"=w167, "Action Name"="Properties Page Edits") -> (w168:T3)
      }
      event "Cancel": Value Change; Panel Close {
        w183 = T19[] [enum."[Data] Legend Strings", enum."[Plot] Data Point", enum."[Plot] Tacho Point", enum."[Plot] Caption", enum."[Plot] Grid and BG", enum."[Axis] Range X Scale", enum."[Axis] Range Y Scale", enum."[Axis] Axis and Label", enum."[Axis] Format String", enum."[Cursor] Appearance", enum."[Cursor] Index", enum."[Cursor] Cursor Info", enum."[Legend] Pair Strings", enum."[Legend] Checkbox", enum."[Legend] Tree Open", enum."[Legend] Color"] items=["None", "[Axis] Range X Scale", "[Axis] Range Y Scale", "[Layout] Graph Type Change", "[Plot] Tacho Point", "[Plot] Grid and BG", "[Cursor] Cursor Info", "[Legend] Pair Strings", "[Data] Plot Data", "[Legend] Checkbox", "[Layout] Update", "[Legend] Tree Open", "[Layout] Legend Visible Change", "[Plot] Data Point", "[Cursor] Appearance", "[Cursor] Index", "[Legend] Color", "[Axis] Axis and Label", "[Axis] Format String", "[Layout] Min Pane Size", "[Data] Index", "[Plot] Caption", "[Data] Legend Strings"]
        n110 = event-data() -> ()  [unwired: 1 in, 1 out]
        n111 = property class="Ctl"(reference=w182) -> (reference out=w181:refnum<vi>, "Desc"=w180:string, "TipStrip"=w179:string, "Label.Text"=w178:string, "Label.Visible"=w177:bool, "Caption.Text"=w176:string, "Caption.Visible"=w175:bool, "Disabled"=w174:u8)  [unwired: 1 in, 1 out]
        n112 = Bundle("Desc"=w180, "TipStrip"=w179, "Label.Text"=w178, "Label.Visible"=w177, "Caption.Text"=w176, "Caption.Visible"=w175, "Disabled"=w174) -> (w173:T17)  [unwired: 1 in]
        n113 = Not Equal?(x=w173, y=w172) -> (x != y?=w171:bool)
        n114 = case shown="True" w171 {
          tunnel: w181 -> [_ w188]
          tunnel: w172 -> [_ w187]
          frame False {
          }
          frame True {
            n115 = Unbundle(w187) -> ("Desc"=w195:string, "TipStrip"=w194:string, "Label.Text"=w193:string, "Label.Visible"=w192:bool, "Caption.Text"=w191:string, "Caption.Visible"=w190:bool, "Disabled"=w189:u8)
            n116 = property class="Ctl"(reference=w188, "Desc"=w195, "TipStrip"=w194, "Label.Text"=w193, "Label.Visible"=w192, "Caption.Text"=w191, "Caption.Visible"=w190, "Disabled"=w189) -> ()  [unwired: 1 in, 2 out]
          }
        }
      }
      event "Help": Value Change {
        n117 = event-data() -> ()  [unwired: 1 in, 6 out]
        n118 = Control Online Help(2:path "<helpdir>/sndvibtk.chm" ("Path to the help file"), 3:"Timebase_Plot_DB.html" ("String to search for"), 4:enum16{"Contents", "Key", "Close"}."Key" ("Operation")) -> ()  [unwired: 1 in, 1 out]
      }
      event "Label.Visible": Value Change {
        n119 = event-data() -> ("NewVal"=w204:bool)  [unwired: 1 in]
        n120 = property class="Ctl"(reference=w207, "Label.Visible"=w204) -> ()  [unwired: 1 in, 2 out]
        n121 = Select(t=u8 0 ("Disabled"), s=w204, f=u8 2) -> (s? t:f=w203:u8)
        n122 = property on="Label.Text" class="Str"("Disabled"=w203) -> ()  [unwired: 2 in, 2 out]
      }
      event "Caption.Visible": Value Change {
        n123 = event-data() -> ("NewVal"=w211:bool)  [unwired: 1 in]
        n124 = property class="Ctl"(reference=w214, "Caption.Visible"=w211) -> ()  [unwired: 1 in, 2 out]
        n125 = Select(t=u8 0 ("Disabled"), s=w211, f=u8 2) -> (s? t:f=w210:u8)
        n126 = property on="Caption.Text" class="Str"("Disabled"=w210) -> ()  [unwired: 2 in, 2 out]
      }
      event "Label.Text": Value Change {
        n127 = event-data() -> ("NewVal"=w217:string)  [unwired: 1 in]
        n128 = property class="Ctl"(reference=w218, "Label.Text"=w217) -> ()  [unwired: 1 in, 2 out]
      }
      event "Caption.Text": Value Change {
        n129 = event-data() -> ("NewVal"=w221:string)  [unwired: 1 in]
        n130 = property class="Ctl"(reference=w222, "Caption.Text"=w221) -> ()  [unwired: 1 in, 2 out]
      }
      event "Enable State": Value Change {
        n131 = event-data() -> ("NewVal"=w225:T9)  [unwired: 1 in]
        n132 = property class="Ctl"(reference=w226, "Disabled"=w225) -> ()  [unwired: 1 in, 2 out]
      }
      event "Background.Color": Value Change {
        w228 = T19[] [enum."[Plot] Grid and BG"] items=["None", "[Axis] Range X Scale", "[Axis] Range Y Scale", "[Layout] Graph Type Change", "[Plot] Tacho Point", "[Plot] Grid and BG", "[Cursor] Cursor Info", "[Legend] Pair Strings", "[Data] Plot Data", "[Legend] Checkbox", "[Layout] Update", "[Legend] Tree Open", "[Layout] Legend Visible Change", "[Plot] Data Point", "[Cursor] Appearance", "[Cursor] Index", "[Legend] Color", "[Axis] Axis and Label", "[Axis] Format String", "[Layout] Min Pane Size", "[Data] Index", "[Plot] Caption", "[Data] Legend Strings"] ("event")
        n133 = event-data() -> ("NewVal"=w229:u32)  [unwired: 1 in]
        n134 = Bundle By Name(cluster=w231, "Background color"=w229) -> (w230:T4)
      }
      event "Digits", "Hide trailing zeros", "Type", "Precision Type": Value Change {
        w233 = T19[] [enum."[Axis] Format String", enum."[Cursor] Cursor Info"] items=["None", "[Axis] Range X Scale", "[Axis] Range Y Scale", "[Layout] Graph Type Change", "[Plot] Tacho Point", "[Plot] Grid and BG", "[Cursor] Cursor Info", "[Legend] Pair Strings", "[Data] Plot Data", "[Legend] Checkbox", "[Layout] Update", "[Legend] Tree Open", "[Layout] Legend Visible Change", "[Plot] Data Point", "[Cursor] Appearance", "[Cursor] Index", "[Legend] Color", "[Axis] Axis and Label", "[Axis] Format String", "[Layout] Min Pane Size", "[Data] Index", "[Plot] Caption", "[Data] Legend Strings"] ("event")
        n135 = event-data() -> ()  [unwired: 1 in, 1 out]
        n136 = call <vilib>:"svx_Timebase To FString.vi"("trailing zeros"="Hide trailing zeros", "Precision Type"="Precision Type", "Digits"="Digits", "Type"="Type") -> ("format string"=w238:string)  [unwired: 7 in]
        n137 = case shown="1" "Format Selection" {
          tunnel: w235 -> [_ _]
          tunnel: w238 -> [w244 w247]
          tunnel: w237 -> [w246 w249]
          tunnel: [w245 w248] -> w236
          tunnel: w234 -> [_ _]
          frame 0, Default {
            n138 = Bundle By Name(cluster=w246, "X Scale.FString"=w244) -> (w245:T4)
          }
          frame 1 {
            n139 = Bundle By Name(cluster=w249, "Y Scale.FString"=w247) -> (w248:T4)
          }
        }
      }
      event "Format Selection": Value Change {
        n140 = event-data() -> ("NewVal"=w257:u16)  [unwired: 1 in]
        n141 = case shown="0, Default" w257 {
          tunnel: w256 -> [w259 w261]
          tunnel: [w258 w260] -> w255
          frame 0, Default {
            n142 = Unbundle By Name(w259) -> ("X Scale.FString"=w258:string)
          }
          frame 1 {
            n143 = Unbundle By Name(w261) -> ("Y Scale.FString"=w260:string)
          }
        }
        n144 = call <vilib>:"svx_Timebase From FString.vi"("Format string"=w255) -> ("trailing zeros"=w251:bool, "Precision Type"=w252:u16, "Digits"=w253:u8, "Type"=w254:i32)  [unwired: 7 in]
        n145 = local write "Hide trailing zeros"(w251) -> ()
        n146 = local write "Precision Type"(w252) -> ()
        n147 = local write "Digits"(w253) -> ()
        n148 = local write "Type"(w254) -> ()
      }
      event "Plot.Line Style": Value Change {
        w263 = T19[] [enum."[Plot] Data Point"] items=["None", "[Axis] Range X Scale", "[Axis] Range Y Scale", "[Layout] Graph Type Change", "[Plot] Tacho Point", "[Plot] Grid and BG", "[Cursor] Cursor Info", "[Legend] Pair Strings", "[Data] Plot Data", "[Legend] Checkbox", "[Layout] Update", "[Legend] Tree Open", "[Layout] Legend Visible Change", "[Plot] Data Point", "[Cursor] Appearance", "[Cursor] Index", "[Legend] Color", "[Axis] Axis and Label", "[Axis] Format String", "[Layout] Min Pane Size", "[Data] Index", "[Plot] Caption", "[Data] Legend Strings"] ("event")
        w272 = bool[] []
        n149 = event-data() -> ("CtlRef"=w267:refnum<vi>, "OldVal"=w273:T11, "NewVal"=w274:T11)  [unwired: 1 in]
        n150 = Variant To Data(type=w272, Variant=w274) -> (data=w271:bool[])  [unwired: 1 in, 1 out]
        n151 = Variant To Data(type=w272, Variant=w273) -> (data=w270:bool[])  [unwired: 1 in, 1 out]
        n152 = Exclusive Or(1:w271, 2:w270) -> (0:w269:bool[])
        n153 = Search 1D Array(1D array=w269, element=TRUE) -> (index of element=w264:i32)  [unwired: 1 in]
        n154 = Bundle By Name(cluster=w266, "Plot.Line Style"=w264) -> (w265:T4)
        n155 = call <vilib>:"svx_Timebase Manage Cluster.vi"("index"=w264, "Cursor Refnum"=w267) -> ()  [unwired: 10 in]
      }
      event "Plot.Line Width": Value Change {
        w276 = T19[] [enum."[Plot] Data Point"] items=["None", "[Axis] Range X Scale", "[Axis] Range Y Scale", "[Layout] Graph Type Change", "[Plot] Tacho Point", "[Plot] Grid and BG", "[Cursor] Cursor Info", "[Legend] Pair Strings", "[Data] Plot Data", "[Legend] Checkbox", "[Layout] Update", "[Legend] Tree Open", "[Layout] Legend Visible Change", "[Plot] Data Point", "[Cursor] Appearance", "[Cursor] Index", "[Legend] Color", "[Axis] Axis and Label", "[Axis] Format String", "[Layout] Min Pane Size", "[Data] Index", "[Plot] Caption", "[Data] Legend Strings"] ("event")
        w287 = bool[] []
        n156 = event-data() -> ("CtlRef"=w278:refnum<vi>, "OldVal"=w279:T12, "NewVal"=w280:T12)  [unwired: 1 in]
        n157 = Variant To Data(type=w287, Variant=w280) -> (data=w286:bool[])  [unwired: 1 in, 1 out]
        n158 = Variant To Data(type=w287, Variant=w279) -> (data=w285:bool[])  [unwired: 1 in, 1 out]
        n159 = Exclusive Or(1:w286, 2:w285) -> (0:w284:bool[])
        n160 = Search 1D Array(1D array=w284, element=TRUE) -> (index of element=w277:i32)  [unwired: 1 in]
        n161 = Bundle By Name(cluster=w282, "Plot.Line Width"=w277) -> (w281:T4)
        n162 = call <vilib>:"svx_Timebase Manage Cluster.vi"("index"=w277, "Cursor Refnum"=w278) -> ()  [unwired: 10 in]
      }
      event "Plot.Point Style": Value Change {
        w289 = T19[] [enum."[Plot] Data Point"] items=["None", "[Axis] Range X Scale", "[Axis] Range Y Scale", "[Layout] Graph Type Change", "[Plot] Tacho Point", "[Plot] Grid and BG", "[Cursor] Cursor Info", "[Legend] Pair Strings", "[Data] Plot Data", "[Legend] Checkbox", "[Layout] Update", "[Legend] Tree Open", "[Layout] Legend Visible Change", "[Plot] Data Point", "[Cursor] Appearance", "[Cursor] Index", "[Legend] Color", "[Axis] Axis and Label", "[Axis] Format String", "[Layout] Min Pane Size", "[Data] Index", "[Plot] Caption", "[Data] Legend Strings"] ("event")
        w300 = bool[] []
        n163 = event-data() -> ("CtlRef"=w291:refnum<vi>, "OldVal"=w292:T10, "NewVal"=w293:T10)  [unwired: 1 in]
        n164 = Variant To Data(type=w300, Variant=w293) -> (data=w299:bool[])  [unwired: 1 in, 1 out]
        n165 = Variant To Data(type=w300, Variant=w292) -> (data=w298:bool[])  [unwired: 1 in, 1 out]
        n166 = Exclusive Or(1:w299, 2:w298) -> (0:w297:bool[])
        n167 = Search 1D Array(1D array=w297, element=TRUE) -> (index of element=w290:i32)  [unwired: 1 in]
        n168 = Bundle By Name(cluster=w295, "Plot.Point Style"=w290) -> (w294:T4)
        n169 = call <vilib>:"svx_Timebase Manage Cluster.vi"("index"=w290, "Cursor Refnum"=w291) -> ()  [unwired: 10 in]
      }
      event "Line.Color": Value Change {
        w302 = T19[] [enum."[Plot] Data Point"] items=["None", "[Axis] Range X Scale", "[Axis] Range Y Scale", "[Layout] Graph Type Change", "[Plot] Tacho Point", "[Plot] Grid and BG", "[Cursor] Cursor Info", "[Legend] Pair Strings", "[Data] Plot Data", "[Legend] Checkbox", "[Layout] Update", "[Legend] Tree Open", "[Layout] Legend Visible Change", "[Plot] Data Point", "[Cursor] Appearance", "[Cursor] Index", "[Legend] Color", "[Axis] Axis and Label", "[Axis] Format String", "[Layout] Min Pane Size", "[Data] Index", "[Plot] Caption", "[Data] Legend Strings"] ("event")
        n170 = event-data() -> ("NewVal"=w303:u32)  [unwired: 1 in]
        n171 = Bundle By Name(cluster=w305, "Plot.Plot Color"=w303) -> (w304:T4)
      }
      event "Trigger Point.Color": Value Change {
        w307 = T19[] [enum."[Plot] Tacho Point"] items=["None", "[Axis] Range X Scale", "[Axis] Range Y Scale", "[Layout] Graph Type Change", "[Plot] Tacho Point", "[Plot] Grid and BG", "[Cursor] Cursor Info", "[Legend] Pair Strings", "[Data] Plot Data", "[Legend] Checkbox", "[Layout] Update", "[Legend] Tree Open", "[Layout] Legend Visible Change", "[Plot] Data Point", "[Cursor] Appearance", "[Cursor] Index", "[Legend] Color", "[Axis] Axis and Label", "[Axis] Format String", "[Layout] Min Pane Size", "[Data] Index", "[Plot] Caption", "[Data] Legend Strings"] ("event")
        n172 = event-data() -> ("NewVal"=w309:u32)  [unwired: 1 in]
        n173 = Bundle By Name(cluster=w310, "Tacho Point Color"=w309) -> (w308:T4)
      }
      event "Cursor.Visible": Value Change {
        w312 = T19[] [enum."[Cursor] Cursor Info"] items=["None", "[Axis] Range X Scale", "[Axis] Range Y Scale", "[Layout] Graph Type Change", "[Plot] Tacho Point", "[Plot] Grid and BG", "[Cursor] Cursor Info", "[Legend] Pair Strings", "[Data] Plot Data", "[Legend] Checkbox", "[Layout] Update", "[Legend] Tree Open", "[Layout] Legend Visible Change", "[Plot] Data Point", "[Cursor] Appearance", "[Cursor] Index", "[Legend] Color", "[Axis] Axis and Label", "[Axis] Format String", "[Layout] Min Pane Size", "[Data] Index", "[Plot] Caption", "[Data] Legend Strings"] ("event")
        n174 = event-data() -> ("NewVal"=w317:bool)  [unwired: 1 in]
        n175 = Unbundle By Name(w319) -> ("Cursor.Cursor Name Visible"=w318:bool)
        n176 = And(x=w317, y=w318) -> (x .and. y?=w314:bool)
        n177 = Select(t=u8 0, s=w317, f=u8 2) -> (s? t:f=w320:u8)
        n178 = Bundle By Name(cluster=w319, "Cursor.Cursor Visible"=w317) -> (w323:T4)
        n179 = Select(t=u8 0, s=w314, f=u8 2) -> (s? t:f=w313:u8)
        n180 = property on="Cursor Info.Visible" class="Bool (strict)"("Disabled"=w320) -> ()  [unwired: 2 in, 2 out]
        n181 = property on="Cursor Info Position.Lock" class="Bool (strict)"("Disabled"=w313) -> ()  [unwired: 2 in, 2 out]
      }
      event "Description": Value Change {
        n182 = event-data() -> ("NewVal"=w326:string)  [unwired: 1 in]
        n183 = property class="Ctl"(reference=w327, "Desc"=w326) -> ()  [unwired: 1 in, 2 out]
      }
      event "Tip strip": Value Change {
        n184 = event-data() -> ("NewVal"=w330:string)  [unwired: 1 in]
        n185 = property class="Ctl"(reference=w331, "TipStrip"=w330) -> ()  [unwired: 1 in, 2 out]
      }
      event "Scale Name": Value Change {
        w333 = T19[] [enum."[Axis] Axis and Label"] items=["None", "[Axis] Range X Scale", "[Axis] Range Y Scale", "[Layout] Graph Type Change", "[Plot] Tacho Point", "[Plot] Grid and BG", "[Cursor] Cursor Info", "[Legend] Pair Strings", "[Data] Plot Data", "[Legend] Checkbox", "[Layout] Update", "[Legend] Tree Open", "[Layout] Legend Visible Change", "[Plot] Data Point", "[Cursor] Appearance", "[Cursor] Index", "[Legend] Color", "[Axis] Axis and Label", "[Axis] Format String", "[Layout] Min Pane Size", "[Data] Index", "[Plot] Caption", "[Data] Legend Strings"] ("event")
        n186 = event-data() -> ("NewVal"=w337:string)  [unwired: 1 in]
        n187 = local read "Scale Selection"() -> (w334:u16)
        n188 = case shown="1" w334 {
          tunnel: w337 -> [w338 w346]
          tunnel: w336 -> [w345 w353]
          tunnel: [w344 w352] -> w335
          frame 0, Default {
            n189 = Bundle By Name(cluster=w345, "X Scale.Name"=w338) -> (w344:T4)
            n190 = property on="Format Selection" class="Ring (strict)"() -> ("Strings []"=w342:string[])  [unwired: 2 in, 2 out]
            n191 = Concatenate Strings(w338, " (X-Axis)" ("string")) -> (w341:string)
            n192 = Replace Array Subset(array=w342, new element=w341, index=0) -> (w339:string[])
            n193 = property on="Format Selection" class="Ring (strict)"("Strings []"=w339) -> ()  [unwired: 2 in, 2 out]
            n194 = property on="Scale Selection" class="Ring (strict)"("Strings []"=w339) -> ()  [unwired: 2 in, 2 out]
          }
          frame 1 {
            n195 = Bundle By Name(cluster=w353, "Y Scale.Name"=w346) -> (w352:T4)
            n196 = property on="Format Selection" class="Ring (strict)"() -> ("Strings []"=w350:string[])  [unwired: 2 in, 2 out]
            n197 = Concatenate Strings(w346, " (Y-Axis)" ("string")) -> (w349:string)
            n198 = Replace Array Subset(array=w350, new element=w349, index=1) -> (w347:string[])
            n199 = property on="Format Selection" class="Ring (strict)"("Strings []"=w347) -> ()  [unwired: 2 in, 2 out]
            n200 = property on="Scale Selection" class="Ring (strict)"("Strings []"=w347) -> ()  [unwired: 2 in, 2 out]
          }
        }
      }
      event "Y Axis Scale": Value Change {
        w355 = T19[] [enum."[Axis] Axis and Label"] items=["None", "[Axis] Range X Scale", "[Axis] Range Y Scale", "[Layout] Graph Type Change", "[Plot] Tacho Point", "[Plot] Grid and BG", "[Cursor] Cursor Info", "[Legend] Pair Strings", "[Data] Plot Data", "[Legend] Checkbox", "[Layout] Update", "[Legend] Tree Open", "[Layout] Legend Visible Change", "[Plot] Data Point", "[Cursor] Appearance", "[Cursor] Index", "[Legend] Color", "[Axis] Axis and Label", "[Axis] Format String", "[Layout] Min Pane Size", "[Data] Index", "[Plot] Caption", "[Data] Legend Strings"] ("event")
        n201 = event-data() -> ("NewVal.Scale Visible"=w356:bool, "NewVal.Scale Label Visible"=w357:bool)  [unwired: 1 in]
        n202 = Bundle By Name(cluster=w359, "Y Scale.Scale Visible"=w356, "Y Scale.Label Visible"=w357) -> (w358:T4)
      }
      event "Scale Fit": Value Change {
        n203 = event-data() -> ("NewVal"=w367:bool)  [unwired: 1 in]
        n204 = local read "Scale Selection"() -> (w363:u16)
        n205 = Boolean To (0,1)(Boolean=w367) -> (0, 1=w366:i16)
        n206 = Add(x=w366, y=w366) -> (x+y=w361:i16)
        n207 = case shown="0, Default" w363 {
          tunnel: w369 -> [w382 w400]
          tunnel: w368 -> [w381 w399]
          tunnel: w367 -> [w380 w398]
          tunnel: [w377 w395] -> w365
          tunnel: w364 -> [w371 w394]
          tunnel: w362 -> [w379 w397]
          tunnel: w361 -> [w372 w385]
          frame 0, Default {
            n208 = Unbundle By Name(w371) -> ("reference"=w370:dbl[])
            n209 = property on="X Axis Range" class="Clust (strict)"("Disabled"=w372) -> ("Controls[]"=w373:refnum<vi>[])  [unwired: 2 in, 2 out]
            n210 = Bundle By Name(cluster=w381, "X Scale.Autoscale"=w380) -> (w378:T4)
            n211 = for {
              tunnel: w373 -> [w384] mode=indexing
              tunnel: w372 -> [w383]
              n212 = property class="Ctl"(reference=w384, "Disabled"=w383) -> ()  [unwired: 1 in, 2 out]
            }
            n213 = call <vilib>:"svx_Timebase Autoscale X.vi"("State In"=w378, "Time Ref"=w370, "Probe Y"=w379, "Probe X"=w382) -> ("State Out"=w377:T4)  [unwired: 7 in]
            n214 = Unbundle By Name(w377) -> ("X Scale.Minimum"=w376:dbl, "X Scale.Maximum"=w375:dbl)
            n215 = Bundle("Minimum"=w376, "Maximum"=w375) -> (w374:cluster{"Minimum":dbl, "Maximum":dbl})  [unwired: 1 in]
            n216 = local write "X Axis Range"(w374) -> ()
          }
          frame 1 {
            n217 = Unbundle By Name(w394) -> ("Y"=w392:dbl[], "X"=w393:dbl[])
            n218 = property on="Y Axis Range" class="Clust (strict)"("Disabled"=w385) -> ("Controls[]"=w386:refnum<vi>[])  [unwired: 2 in, 2 out]
            n219 = Bundle By Name(cluster=w399, "Y Scale.Autoscale"=w398) -> (w396:T4)
            n220 = for {
              tunnel: w386 -> [w402] mode=indexing
              tunnel: w385 -> [w401]
              n221 = property class="Ctl"(reference=w402, "Disabled"=w401) -> ()  [unwired: 1 in, 2 out]
            }
            n222 = call <vilib>:"svx_Timebase Autoscale Y.vi"("Y"=w392, "State In"=w396, "X"=w393, "Probe Y"=w397, "Probe X"=w400) -> ("State Out"=w395:T4)  [unwired: 6 in]
            n223 = Unbundle By Name(w395) -> ("Y Scale.Minimum.Probe X"=w391:dbl, "Y Scale.Maximum.Probe X"=w390:dbl, "Y Scale.Minimum.Probe Y"=w389:dbl, "Y Scale.Maximum.Probe Y"=w388:dbl)
            n224 = Bundle("Probe X"=w391, "Probe X"=w390, "Probe Y"=w389, "Probe Y"=w388) -> (w387:T20)  [unwired: 1 in]
            n225 = local write "Y Axis Range"(w387) -> ()
          }
        }
      }
      event "X Axis Range": Value Change {
        w404 = T19[] [enum."[Axis] Range X Scale"] items=["None", "[Axis] Range X Scale", "[Axis] Range Y Scale", "[Layout] Graph Type Change", "[Plot] Tacho Point", "[Plot] Grid and BG", "[Cursor] Cursor Info", "[Legend] Pair Strings", "[Data] Plot Data", "[Legend] Checkbox", "[Layout] Update", "[Legend] Tree Open", "[Layout] Legend Visible Change", "[Plot] Data Point", "[Cursor] Appearance", "[Cursor] Index", "[Legend] Color", "[Axis] Axis and Label", "[Axis] Format String", "[Layout] Min Pane Size", "[Data] Index", "[Plot] Caption", "[Data] Legend Strings"] ("event")
        n226 = event-data() -> ("NewVal.Minimum X"=w409:dbl, "NewVal.Maximum X"=w408:dbl)  [unwired: 1 in]
        n227 = Max & Min(x=w409, y=w408) -> (max(x,y)=w406:dbl, min(x,y)=w407:dbl)
        n228 = Bundle(w407, w406) -> (w405:cluster{dbl, dbl})  [unwired: 1 in]
        n229 = Bundle By Name(cluster=w411, "X Scale.Maximum"=w406, "X Scale.Minimum"=w407) -> (w410:T4)
        n230 = local write "X Axis Range"(w405) -> ()
      }
      event "XGrid Style": Value Change {
        w416 = T19[] [enum."[Plot] Grid and BG"] items=["None", "[Axis] Range X Scale", "[Axis] Range Y Scale", "[Layout] Graph Type Change", "[Plot] Tacho Point", "[Plot] Grid and BG", "[Cursor] Cursor Info", "[Legend] Pair Strings", "[Data] Plot Data", "[Legend] Checkbox", "[Layout] Update", "[Legend] Tree Open", "[Layout] Legend Visible Change", "[Plot] Data Point", "[Cursor] Appearance", "[Cursor] Index", "[Legend] Color", "[Axis] Axis and Label", "[Axis] Format String", "[Layout] Min Pane Size", "[Data] Index", "[Plot] Caption", "[Data] Legend Strings"] ("event")
        n231 = event-data() -> ("NewVal"=w413:u16)  [unwired: 1 in]
        n232 = case shown="1" w413 {
          tunnel: [w419 u8 0 ("Disabled") w422] -> w414
          tunnel: [w419 u8 2 ("Disabled") w422] -> w415
          frame 0, Default {
            w419 = u8 2 ("Disabled")
          }
          frame 1 {
          }
          frame 2 {
            w422 = u8 0 ("Disabled")
          }
        }
        n233 = property on="Major Grid.Color" class="ColBox"("Disabled"=w414) -> ()  [unwired: 2 in, 2 out]
        n234 = property on="Minor Grid.Color" class="ColBox"("Disabled"=w415) -> ()  [unwired: 2 in, 2 out]
        n235 = Bundle By Name(cluster=w417, "X Scale.Grid Style"=w413) -> (w418:T4)
      }
      event "YGrid Style": Value Change {
        w427 = T19[] [enum."[Plot] Grid and BG"] items=["None", "[Axis] Range X Scale", "[Axis] Range Y Scale", "[Layout] Graph Type Change", "[Plot] Tacho Point", "[Plot] Grid and BG", "[Cursor] Cursor Info", "[Legend] Pair Strings", "[Data] Plot Data", "[Legend] Checkbox", "[Layout] Update", "[Legend] Tree Open", "[Layout] Legend Visible Change", "[Plot] Data Point", "[Cursor] Appearance", "[Cursor] Index", "[Legend] Color", "[Axis] Axis and Label", "[Axis] Format String", "[Layout] Min Pane Size", "[Data] Index", "[Plot] Caption", "[Data] Legend Strings"] ("event")
        n236 = event-data() -> ("NewVal"=w424:u16)  [unwired: 1 in]
        n237 = case shown="1" w424 {
          tunnel: [w430 u8 0 ("Disabled") w433] -> w425
          tunnel: [w430 u8 2 ("Disabled") w433] -> w426
          frame 0, Default {
            w430 = u8 2 ("Disabled")
          }
          frame 1 {
          }
          frame 2 {
            w433 = u8 0 ("Disabled")
          }
        }
        n238 = property on="Major Grid.Color" class="ColBox"("Disabled"=w425) -> ()  [unwired: 2 in, 2 out]
        n239 = property on="Minor Grid.Color" class="ColBox"("Disabled"=w426) -> ()  [unwired: 2 in, 2 out]
        n240 = Bundle By Name(cluster=w428, "Y Scale.Grid Style"=w424) -> (w429:T4)
      }
      event "Major Grid.Color": Value Change {
        w435 = T19[] [enum."[Plot] Grid and BG"] items=["None", "[Axis] Range X Scale", "[Axis] Range Y Scale", "[Layout] Graph Type Change", "[Plot] Tacho Point", "[Plot] Grid and BG", "[Cursor] Cursor Info", "[Legend] Pair Strings", "[Data] Plot Data", "[Legend] Checkbox", "[Layout] Update", "[Legend] Tree Open", "[Layout] Legend Visible Change", "[Plot] Data Point", "[Cursor] Appearance", "[Cursor] Index", "[Legend] Color", "[Axis] Axis and Label", "[Axis] Format String", "[Layout] Min Pane Size", "[Data] Index", "[Plot] Caption", "[Data] Legend Strings"] ("event")
        n241 = event-data() -> ("NewVal"=w437:u32)  [unwired: 1 in]
        n242 = local read "Scale Selection"() -> (w436:u16)
        n243 = case shown="0, Default" w436 {
          tunnel: w439 -> [w442 w445]
          tunnel: [w441 w444] -> w438
          tunnel: w437 -> [w440 w443]
          frame 0, Default {
            n244 = Bundle By Name(cluster=w442, "X Scale.Major Color"=w440) -> (w441:T4)
          }
          frame 1 {
            n245 = Bundle By Name(cluster=w445, "Y Scale.Major Color"=w443) -> (w444:T4)
          }
        }
      }
      event "Minor Grid.Color": Value Change {
        w447 = T19[] [enum."[Plot] Grid and BG"] items=["None", "[Axis] Range X Scale", "[Axis] Range Y Scale", "[Layout] Graph Type Change", "[Plot] Tacho Point", "[Plot] Grid and BG", "[Cursor] Cursor Info", "[Legend] Pair Strings", "[Data] Plot Data", "[Legend] Checkbox", "[Layout] Update", "[Legend] Tree Open", "[Layout] Legend Visible Change", "[Plot] Data Point", "[Cursor] Appearance", "[Cursor] Index", "[Legend] Color", "[Axis] Axis and Label", "[Axis] Format String", "[Layout] Min Pane Size", "[Data] Index", "[Plot] Caption", "[Data] Legend Strings"] ("event")
        n246 = event-data() -> ("NewVal"=w449:u32)  [unwired: 1 in]
        n247 = local read "Scale Selection"() -> (w448:u16)
        n248 = case shown="1" w448 {
          tunnel: w451 -> [w454 w457]
          tunnel: [w453 w456] -> w450
          tunnel: w449 -> [w452 w455]
          frame 0, Default {
            n249 = Bundle By Name(cluster=w454, "X Scale.Minor Color"=w452) -> (w453:T4)
          }
          frame 1 {
            n250 = Bundle By Name(cluster=w457, "Y Scale.Minor Color"=w455) -> (w456:T4)
          }
        }
      }
      event "Scale Selection": Value Change {
        n251 = event-data() -> ("NewVal"=w466:u16)  [unwired: 1 in]
        n252 = case shown="1" w466 {
          tunnel: [w478 w498] -> w470
          tunnel: [w490 w510] -> w469
          tunnel: [w489 w509] -> w468
          tunnel: [w488 w508] -> w463
          tunnel: [w487 w507] -> w462
          tunnel: [w486 w506] -> w467
          tunnel: w465 -> [w485 w505]
          tunnel: [w482 w502] -> w464
          tunnel: [FALSE ("Visible") TRUE ("Visible")] -> w459
          tunnel: [TRUE ("Visible") FALSE ("Visible")] -> w460
          frame 0, Default {
            n253 = Unbundle By Name(w485) -> ("X Scale.Name"=w486:string, "X Scale.Show Scale Label.Probe X"=w487:bool, "Y Scale.Scale Visible"=w488:bool, "X Scale.Major Color"=w489:u32, "X Scale.Minor Color"=w490:u32, "X Scale.Autoscale"=w478:bool, "X Scale.Minimum"=w475:dbl, "X Scale.Maximum"=w474:dbl, "X Scale.Grid Style"=w482:u16)
            n254 = local write "XGrid Style"(w482) -> ()
            n255 = property on="XGrid Style" class="Ring (strict)"("Visible"=TRUE) -> ()  [unwired: 2 in, 2 out]
            n256 = property on="YGrid Style" class="Ring (strict)"("Visible"=FALSE) -> ()  [unwired: 2 in, 2 out]
            n257 = Bundle("Minimum"=w475, "Maximum"=w474) -> (w473:cluster{"Minimum":dbl, "Maximum":dbl})  [unwired: 1 in]
            n258 = Select(t=u8 2 ("Disabled"), s=w478, f=u8 0) -> (s? t:f=w479:u8)
            n259 = local write "X Axis Range"(w473) -> ()
            n260 = property on="X Axis Range" class="Clust (strict)"("Disabled"=w479) -> ()  [unwired: 2 in, 2 out]
          }
          frame 1 {
            n261 = Unbundle By Name(w505) -> ("Y Scale.Name"=w506:string, "Y Scale.Scale Visible"=w507:bool, "Y Scale.Label Visible"=w508:bool, "Y Scale.Major Color"=w509:u32, "Y Scale.Minor Color"=w510:u32, "Y Scale.Autoscale"=w498:bool, "Y Scale.Minimum.Probe X"=w495:dbl, "Y Scale.Maximum.Probe X"=w494:dbl, "Y Scale.Minimum.Probe Y"=w493:dbl, "Y Scale.Maximum.Probe Y"=w492:dbl, "Y Scale.Grid Style"=w502:u16)
            n262 = property on="XGrid Style" class="Ring (strict)"("Visible"=FALSE) -> ()  [unwired: 2 in, 2 out]
            n263 = local write "YGrid Style"(w502) -> ()
            n264 = property on="YGrid Style" class="Ring (strict)"("Visible"=TRUE) -> ()  [unwired: 2 in, 2 out]
            n265 = Select(t=u8 2 ("Disabled"), s=w498, f=u8 0) -> (s? t:f=w499:u8)
            n266 = Bundle("Probe X"=w495, "Probe X"=w494, "Probe Y"=w493, "Probe Y"=w492) -> (w491:T20)  [unwired: 1 in]
            n267 = property on="Y Axis Range" class="Clust (strict)"("Disabled"=w499) -> ()  [unwired: 2 in, 2 out]
            n268 = local write "Y Axis Range"(w491) -> ()
          }
        }
        n269 = local write "Scale Name"(w467) -> ()
        n270 = local write "Minor Grid.Color"(w469) -> ()
        n271 = Bundle("Scale Visible"=w462, "Label Visible"=w463) -> (w461:T21)  [unwired: 1 in]
        n272 = case shown="1" w464 {
          tunnel: [w511 u8 0 ("Disabled") w514] -> w471
          tunnel: [w511 u8 2 ("Disabled") w514] -> w472
          frame 0, Default {
            w511 = u8 2 ("Disabled")
          }
          frame 1 {
          }
          frame 2 {
            w514 = u8 0 ("Disabled")
          }
        }
        n273 = local write "Y Axis Scale"(w461) -> ()
        n274 = property on="X Axis Range" class="Clust (strict)"("Visible"=w460) -> ()  [unwired: 2 in, 2 out]
        n275 = property on="Y Axis Range" class="Clust (strict)"("Visible"=w459) -> ()  [unwired: 2 in, 2 out]
        n276 = local write "Major Grid.Color"(w468) -> ()
        n277 = local write "Scale Fit"(w470) -> ()
        n278 = property on="X Axis Scale" class="Clust (strict)"("Visible"=w460) -> ()  [unwired: 2 in, 2 out]
        n279 = property on="Y Axis Scale" class="Clust (strict)"("Visible"=w459) -> ()  [unwired: 2 in, 2 out]
        n280 = property on="Major Grid.Color" class="ColBox"("Disabled"=w471) -> ()  [unwired: 2 in, 2 out]
        n281 = property on="Minor Grid.Color" class="ColBox"("Disabled"=w472) -> ()  [unwired: 2 in, 2 out]
      }
      event "Cursor.Line Style": Value Change {
        w516 = T19[] [enum."[Cursor] Appearance"] items=["None", "[Axis] Range X Scale", "[Axis] Range Y Scale", "[Layout] Graph Type Change", "[Plot] Tacho Point", "[Plot] Grid and BG", "[Cursor] Cursor Info", "[Legend] Pair Strings", "[Data] Plot Data", "[Legend] Checkbox", "[Layout] Update", "[Legend] Tree Open", "[Layout] Legend Visible Change", "[Plot] Data Point", "[Cursor] Appearance", "[Cursor] Index", "[Legend] Color", "[Axis] Axis and Label", "[Axis] Format String", "[Layout] Min Pane Size", "[Data] Index", "[Plot] Caption", "[Data] Legend Strings"] ("event")
        w527 = bool[] []
        n282 = event-data() -> ("CtlRef"=w518:refnum<vi>, "OldVal"=w519:T11, "NewVal"=w520:T11)  [unwired: 1 in]
        n283 = Variant To Data(type=w527, Variant=w520) -> (data=w526:bool[])  [unwired: 1 in, 1 out]
        n284 = Variant To Data(type=w527, Variant=w519) -> (data=w525:bool[])  [unwired: 1 in, 1 out]
        n285 = Exclusive Or(1:w526, 2:w525) -> (0:w524:bool[])
        n286 = Search 1D Array(1D array=w524, element=TRUE) -> (index of element=w517:i32)  [unwired: 1 in]
        n287 = Bundle By Name(cluster=w522, "Cursor.Cursor Line Style"=w517) -> (w521:T4)
        n288 = call <vilib>:"svx_Timebase Manage Cluster.vi"("index"=w517, "Cursor Refnum"=w518) -> ()  [unwired: 10 in]
      }
      event "Cursor.Line Width": Value Change {
        w529 = T19[] [enum."[Cursor] Appearance"] items=["None", "[Axis] Range X Scale", "[Axis] Range Y Scale", "[Layout] Graph Type Change", "[Plot] Tacho Point", "[Plot] Grid and BG", "[Cursor] Cursor Info", "[Legend] Pair Strings", "[Data] Plot Data", "[Legend] Checkbox", "[Layout] Update", "[Legend] Tree Open", "[Layout] Legend Visible Change", "[Plot] Data Point", "[Cursor] Appearance", "[Cursor] Index", "[Legend] Color", "[Axis] Axis and Label", "[Axis] Format String", "[Layout] Min Pane Size", "[Data] Index", "[Plot] Caption", "[Data] Legend Strings"] ("event")
        w540 = bool[] []
        n289 = event-data() -> ("CtlRef"=w531:refnum<vi>, "OldVal"=w532:T12, "NewVal"=w533:T12)  [unwired: 1 in]
        n290 = Variant To Data(type=w540, Variant=w533) -> (data=w539:bool[])  [unwired: 1 in, 1 out]
        n291 = Variant To Data(type=w540, Variant=w532) -> (data=w538:bool[])  [unwired: 1 in, 1 out]
        n292 = Exclusive Or(1:w539, 2:w538) -> (0:w537:bool[])
        n293 = Search 1D Array(1D array=w537, element=TRUE) -> (index of element=w530:i32)  [unwired: 1 in]
        n294 = Bundle By Name(cluster=w535, "Cursor.Cursor Line Width"=w530) -> (w534:T4)
        n295 = call <vilib>:"svx_Timebase Manage Cluster.vi"("index"=w530, "Cursor Refnum"=w531) -> ()  [unwired: 10 in]
      }
      event "Cursor.Point Style": Value Change {
        w542 = T19[] [enum."[Cursor] Appearance"] items=["None", "[Axis] Range X Scale", "[Axis] Range Y Scale", "[Layout] Graph Type Change", "[Plot] Tacho Point", "[Plot] Grid and BG", "[Cursor] Cursor Info", "[Legend] Pair Strings", "[Data] Plot Data", "[Legend] Checkbox", "[Layout] Update", "[Legend] Tree Open", "[Layout] Legend Visible Change", "[Plot] Data Point", "[Cursor] Appearance", "[Cursor] Index", "[Legend] Color", "[Axis] Axis and Label", "[Axis] Format String", "[Layout] Min Pane Size", "[Data] Index", "[Plot] Caption", "[Data] Legend Strings"] ("event")
        w553 = bool[] []
        n296 = event-data() -> ("CtlRef"=w544:refnum<vi>, "OldVal"=w545:T10, "NewVal"=w546:T10)  [unwired: 1 in]
        n297 = Variant To Data(type=w553, Variant=w546) -> (data=w552:bool[])  [unwired: 1 in, 1 out]
        n298 = Variant To Data(type=w553, Variant=w545) -> (data=w551:bool[])  [unwired: 1 in, 1 out]
        n299 = Exclusive Or(1:w552, 2:w551) -> (0:w550:bool[])
        n300 = Search 1D Array(1D array=w550, element=TRUE) -> (index of element=w543:i32)  [unwired: 1 in]
        n301 = Bundle By Name(cluster=w548, "Cursor.Cursor Point Style"=w543) -> (w547:T4)
        n302 = call <vilib>:"svx_Timebase Manage Cluster.vi"("index"=w543, "Cursor Refnum"=w544) -> ()  [unwired: 10 in]
      }
      event "Cursor.Style": Value Change {
        w555 = T19[] [enum."[Cursor] Appearance"] items=["None", "[Axis] Range X Scale", "[Axis] Range Y Scale", "[Layout] Graph Type Change", "[Plot] Tacho Point", "[Plot] Grid and BG", "[Cursor] Cursor Info", "[Legend] Pair Strings", "[Data] Plot Data", "[Legend] Checkbox", "[Layout] Update", "[Legend] Tree Open", "[Layout] Legend Visible Change", "[Plot] Data Point", "[Cursor] Appearance", "[Cursor] Index", "[Legend] Color", "[Axis] Axis and Label", "[Axis] Format String", "[Layout] Min Pane Size", "[Data] Index", "[Plot] Caption", "[Data] Legend Strings"] ("event")
        w566 = bool[] []
        n303 = event-data() -> ("CtlRef"=w557:refnum<vi>, "OldVal"=w558:T16, "NewVal"=w559:T16)  [unwired: 1 in]
        n304 = Variant To Data(type=w566, Variant=w559) -> (data=w565:bool[])  [unwired: 1 in, 1 out]
        n305 = Variant To Data(type=w566, Variant=w558) -> (data=w564:bool[])  [unwired: 1 in, 1 out]
        n306 = Exclusive Or(1:w565, 2:w564) -> (0:w563:bool[])
        n307 = Search 1D Array(1D array=w563, element=TRUE) -> (index of element=w556:i32)  [unwired: 1 in]
        n308 = Bundle By Name(cluster=w561, "Cursor.Cursor Style"=w556) -> (w560:T4)
        n309 = call <vilib>:"svx_Timebase Manage Cluster.vi"("index"=w556, "Cursor Refnum"=w557) -> ()  [unwired: 10 in]
      }
      event "Cursor Info.Visible": Value Change {
        w568 = T19[] [enum."[Cursor] Cursor Info"] items=["None", "[Axis] Range X Scale", "[Axis] Range Y Scale", "[Layout] Graph Type Change", "[Plot] Tacho Point", "[Plot] Grid and BG", "[Cursor] Cursor Info", "[Legend] Pair Strings", "[Data] Plot Data", "[Legend] Checkbox", "[Layout] Update", "[Legend] Tree Open", "[Layout] Legend Visible Change", "[Plot] Data Point", "[Cursor] Appearance", "[Cursor] Index", "[Legend] Color", "[Axis] Axis and Label", "[Axis] Format String", "[Layout] Min Pane Size", "[Data] Index", "[Plot] Caption", "[Data] Legend Strings"] ("event")
        n310 = event-data() -> ("NewVal"=w569:bool)  [unwired: 1 in]
        n311 = Select(t=u8 0, s=w569, f=u8 2) -> (s? t:f=w572:u8)
        n312 = Bundle By Name(cluster=w574, "Cursor.Cursor Name Visible"=w569) -> (w573:T4)
        n313 = property on="Cursor Info Position.Lock" class="Bool (strict)"("Disabled"=w572) -> ()  [unwired: 2 in, 2 out]
      }
      event "Cursor.Color": Value Change {
        w576 = T19[] [enum."[Cursor] Appearance", enum."[Cursor] Cursor Info"] items=["None", "[Axis] Range X Scale", "[Axis] Range Y Scale", "[Layout] Graph Type Change", "[Plot] Tacho Point", "[Plot] Grid and BG", "[Cursor] Cursor Info", "[Legend] Pair Strings", "[Data] Plot Data", "[Legend] Checkbox", "[Layout] Update", "[Legend] Tree Open", "[Layout] Legend Visible Change", "[Plot] Data Point", "[Cursor] Appearance", "[Cursor] Index", "[Legend] Color", "[Axis] Axis and Label", "[Axis] Format String", "[Layout] Min Pane Size", "[Data] Index", "[Plot] Caption", "[Data] Legend Strings"] ("event")
        n314 = event-data() -> ("NewVal"=w578:u32)  [unwired: 1 in]
        n315 = Bundle By Name(cluster=w579, "Cursor.Cursor Color"=w578) -> (w577:T4)
      }
      event "Cursor Info Position.Lock": Value Change {
        w581 = T19[] [enum."[Cursor] Cursor Info"] items=["None", "[Axis] Range X Scale", "[Axis] Range Y Scale", "[Layout] Graph Type Change", "[Plot] Tacho Point", "[Plot] Grid and BG", "[Cursor] Cursor Info", "[Legend] Pair Strings", "[Data] Plot Data", "[Legend] Checkbox", "[Layout] Update", "[Legend] Tree Open", "[Layout] Legend Visible Change", "[Plot] Data Point", "[Cursor] Appearance", "[Cursor] Index", "[Legend] Color", "[Axis] Axis and Label", "[Axis] Format String", "[Layout] Min Pane Size", "[Data] Index", "[Plot] Caption", "[Data] Legend Strings"] ("event")
        n316 = event-data() -> ("NewVal"=w583:bool)  [unwired: 1 in]
        n317 = Bundle By Name(cluster=w584, "Cursor.Cursor Lock"=w583) -> (w582:T4)
      }
      event "Point/Fill.Color": Value Change {
        w586 = T19[] [enum."[Plot] Data Point"] items=["None", "[Axis] Range X Scale", "[Axis] Range Y Scale", "[Layout] Graph Type Change", "[Plot] Tacho Point", "[Plot] Grid and BG", "[Cursor] Cursor Info", "[Legend] Pair Strings", "[Data] Plot Data", "[Legend] Checkbox", "[Layout] Update", "[Legend] Tree Open", "[Layout] Legend Visible Change", "[Plot] Data Point", "[Cursor] Appearance", "[Cursor] Index", "[Legend] Color", "[Axis] Axis and Label", "[Axis] Format String", "[Layout] Min Pane Size", "[Data] Index", "[Plot] Caption", "[Data] Legend Strings"] ("event")
        n318 = event-data() -> ("NewVal"=w587:u32)  [unwired: 1 in]
        n319 = Bundle By Name(cluster=w589, "Plot.Point/fill"=w587) -> (w588:T4)
      }
      event "Y Axis Range": Value Change {
        w591 = T19[] [enum."[Axis] Range Y Scale"] items=["None", "[Axis] Range X Scale", "[Axis] Range Y Scale", "[Layout] Graph Type Change", "[Plot] Tacho Point", "[Plot] Grid and BG", "[Cursor] Cursor Info", "[Legend] Pair Strings", "[Data] Plot Data", "[Legend] Checkbox", "[Layout] Update", "[Legend] Tree Open", "[Layout] Legend Visible Change", "[Plot] Data Point", "[Cursor] Appearance", "[Cursor] Index", "[Legend] Color", "[Axis] Axis and Label", "[Axis] Format String", "[Layout] Min Pane Size", "[Data] Index", "[Plot] Caption", "[Data] Legend Strings"] ("event")
        n320 = event-data() -> ("NewVal.Minimum Y [Probe X]"=w597:dbl, "NewVal.Maximum Y [Probe X]"=w598:dbl, "NewVal.Minimum Y [Probe Y]"=w600:dbl, "NewVal.Maximum Y [Probe Y]"=w599:dbl)  [unwired: 1 in]
        n321 = Max & Min(x=w597, y=w598) -> (max(x,y)=w595:dbl, min(x,y)=w596:dbl)
        n322 = Max & Min(x=w600, y=w599) -> (max(x,y)=w593:dbl, min(x,y)=w594:dbl)
        n323 = Bundle By Name(cluster=w602, "Y Scale.Maximum.Probe X"=w595, "Y Scale.Minimum.Probe X"=w596, "Y Scale.Maximum.Probe Y"=w593, "Y Scale.Minimum.Probe Y"=w594) -> (w601:T4)
        n324 = Bundle(w596, w595, w594, w593) -> (w592:cluster{dbl, dbl, dbl, dbl})  [unwired: 1 in]
        n325 = local write "Y Axis Range"(w592) -> ()
      }
      event "X Axis Scale": Value Change {
        w604 = T19[] [enum."[Axis] Axis and Label"] items=["None", "[Axis] Range X Scale", "[Axis] Range Y Scale", "[Layout] Graph Type Change", "[Plot] Tacho Point", "[Plot] Grid and BG", "[Cursor] Cursor Info", "[Legend] Pair Strings", "[Data] Plot Data", "[Legend] Checkbox", "[Layout] Update", "[Legend] Tree Open", "[Layout] Legend Visible Change", "[Plot] Data Point", "[Cursor] Appearance", "[Cursor] Index", "[Legend] Color", "[Axis] Axis and Label", "[Axis] Format String", "[Layout] Min Pane Size", "[Data] Index", "[Plot] Caption", "[Data] Legend Strings"] ("event")
        n326 = event-data() -> ("NewVal.Probe Y Scale.Visible"=w606:bool, "NewVal.Probe Y Scale Label.Visible"=w607:bool, "NewVal.Probe X Scale.Visible"=w605:bool, "NewVal.Probe X Scale Label.Visible"=w608:bool)  [unwired: 1 in]
        n327 = Bundle By Name(cluster=w610, "X Scale.Show Scale.Probe Y"=w606, "X Scale.Show Scale Label.Probe Y"=w607, "X Scale.Show Scale.Probe X"=w605, "X Scale.Show Scale Label.Probe X"=w608) -> (w609:T4)
      }
      event "Probe X Label.Visible": Value Change {
        w612 = T19[] [enum."[Plot] Caption"] items=["None", "[Axis] Range X Scale", "[Axis] Range Y Scale", "[Layout] Graph Type Change", "[Plot] Tacho Point", "[Plot] Grid and BG", "[Cursor] Cursor Info", "[Legend] Pair Strings", "[Data] Plot Data", "[Legend] Checkbox", "[Layout] Update", "[Legend] Tree Open", "[Layout] Legend Visible Change", "[Plot] Data Point", "[Cursor] Appearance", "[Cursor] Index", "[Legend] Color", "[Axis] Axis and Label", "[Axis] Format String", "[Layout] Min Pane Size", "[Data] Index", "[Plot] Caption", "[Data] Legend Strings"] ("event")
        n328 = event-data() -> ("NewVal"=w614:bool)  [unwired: 1 in]
        n329 = Select(t=u8 0 ("Disabled"), s=w614, f=u8 2) -> (s? t:f=w616:u8)
        n330 = property on="Probe X Label.Text" class="Str"("Disabled"=w616) -> ()  [unwired: 2 in, 2 out]
        n331 = Bundle By Name(cluster=w618, "Probe X Label Visible"=w614) -> (w617:T4)
      }
      event "Probe Y Label.Visible": Value Change {
        w620 = T19[] [enum."[Plot] Caption"] items=["None", "[Axis] Range X Scale", "[Axis] Range Y Scale", "[Layout] Graph Type Change", "[Plot] Tacho Point", "[Plot] Grid and BG", "[Cursor] Cursor Info", "[Legend] Pair Strings", "[Data] Plot Data", "[Legend] Checkbox", "[Layout] Update", "[Legend] Tree Open", "[Layout] Legend Visible Change", "[Plot] Data Point", "[Cursor] Appearance", "[Cursor] Index", "[Legend] Color", "[Axis] Axis and Label", "[Axis] Format String", "[Layout] Min Pane Size", "[Data] Index", "[Plot] Caption", "[Data] Legend Strings"] ("event")
        n332 = event-data() -> ("NewVal"=w622:bool)  [unwired: 1 in]
        n333 = Select(t=u8 0 ("Disabled"), s=w622, f=u8 2) -> (s? t:f=w624:u8)
        n334 = property on="Probe Y Label.Text" class="Str"("Disabled"=w624) -> ()  [unwired: 2 in, 2 out]
        n335 = Bundle By Name(cluster=w626, "Probe Y Label Visible"=w622) -> (w625:T4)
      }
      event "Probe X Label.Text": Value Change {
        w628 = T19[] [enum."[Plot] Caption"] items=["None", "[Axis] Range X Scale", "[Axis] Range Y Scale", "[Layout] Graph Type Change", "[Plot] Tacho Point", "[Plot] Grid and BG", "[Cursor] Cursor Info", "[Legend] Pair Strings", "[Data] Plot Data", "[Legend] Checkbox", "[Layout] Update", "[Legend] Tree Open", "[Layout] Legend Visible Change", "[Plot] Data Point", "[Cursor] Appearance", "[Cursor] Index", "[Legend] Color", "[Axis] Axis and Label", "[Axis] Format String", "[Layout] Min Pane Size", "[Data] Index", "[Plot] Caption", "[Data] Legend Strings"] ("event")
        n336 = event-data() -> ("NewVal"=w629:string)  [unwired: 1 in]
        n337 = Bundle By Name(cluster=w631, "Probe X Label"=w629) -> (w630:T4)
      }
      event "Probe Y Label.Text": Value Change {
        w633 = T19[] [enum."[Plot] Caption"] items=["None", "[Axis] Range X Scale", "[Axis] Range Y Scale", "[Layout] Graph Type Change", "[Plot] Tacho Point", "[Plot] Grid and BG", "[Cursor] Cursor Info", "[Legend] Pair Strings", "[Data] Plot Data", "[Legend] Checkbox", "[Layout] Update", "[Legend] Tree Open", "[Layout] Legend Visible Change", "[Plot] Data Point", "[Cursor] Appearance", "[Cursor] Index", "[Legend] Color", "[Axis] Axis and Label", "[Axis] Format String", "[Layout] Min Pane Size", "[Data] Index", "[Plot] Caption", "[Data] Legend Strings"] ("event")
        n338 = event-data() -> ("NewVal"=w634:string)  [unwired: 1 in]
        n339 = Bundle By Name(cluster=w636, "Probe Y Label"=w634) -> (w635:T4)
      }
      event "Legend Background.Color": Value Change {
        w638 = T19[] [enum."[Legend] Color"] items=["None", "[Axis] Range X Scale", "[Axis] Range Y Scale", "[Layout] Graph Type Change", "[Plot] Tacho Point", "[Plot] Grid and BG", "[Cursor] Cursor Info", "[Legend] Pair Strings", "[Data] Plot Data", "[Legend] Checkbox", "[Layout] Update", "[Legend] Tree Open", "[Layout] Legend Visible Change", "[Plot] Data Point", "[Cursor] Appearance", "[Cursor] Index", "[Legend] Color", "[Axis] Axis and Label", "[Axis] Format String", "[Layout] Min Pane Size", "[Data] Index", "[Plot] Caption", "[Data] Legend Strings"] ("event")
        n340 = event-data() -> ("NewVal"=w639:u32)  [unwired: 1 in]
        n341 = Bundle By Name(cluster=w641, "Legend Background"=w639) -> (w640:T4)
      }
      event "Legend Font.Color": Value Change {
        w643 = T19[] [enum."[Legend] Color"] items=["None", "[Axis] Range X Scale", "[Axis] Range Y Scale", "[Layout] Graph Type Change", "[Plot] Tacho Point", "[Plot] Grid and BG", "[Cursor] Cursor Info", "[Legend] Pair Strings", "[Data] Plot Data", "[Legend] Checkbox", "[Layout] Update", "[Legend] Tree Open", "[Layout] Legend Visible Change", "[Plot] Data Point", "[Cursor] Appearance", "[Cursor] Index", "[Legend] Color", "[Axis] Axis and Label", "[Axis] Format String", "[Layout] Min Pane Size", "[Data] Index", "[Plot] Caption", "[Data] Legend Strings"] ("event")
        n342 = event-data() -> ("NewVal"=w646:u32)  [unwired: 1 in]
        n343 = Bundle By Name(cluster=w645, "Legend Font"=w646) -> (w644:T4)
      }
    }
    n344 = call <vilib>:"svx_Timebase Exec Commands.vi"("Display State In"=w153, "Data In"=w154, "Commands"=w147, "Facade VI"=w150, "Ref Ins"=w151, "Container"=w149) -> ("Display State Out"=w152:T4)  [unwired: 5 in]
  }
  "State out" <- w14
  "Action out" <- w17
